vi "Configuration_old.vi"(10 "Open from\nscan VI":bool, 11 "Measurements":T1(tab)) -> (3 "configured?":bool)   [LabVIEW 2013]
uses:
  InstrControl/InstrumentSetup.vi
  InstrControl/InstrControl.lvclass
  globals/QC_MeasurementSetup.vi
  InstrControl/Switching/Switching.lvclass
  globals/QC_RunInformation.vi
panel:
  in  "Defaults Multimeter":bool
  in  "Multimeter":enum32{"Keithley 2000"}(tab)
  in  "Range Value\n(0.1 - 100)":dbl=100.0 format="%#.2g"
  in  "Range":u16(ring) items=["Auto", "Manual"]
  in  "Function":u16(ring)=3 items=["AC Current", "DC Current", "AC Voltage", "DC Voltage", "2W-Resistance", "4W-Resistance", "Period", "Frequency", "Temperature", "Diode", "Continuity"]
  in  "GPIB Address KE2000":i32=19
  in  "Apply":bool
  in  "Defaults LCR":bool
  in  "LCRs":enum32{"WayneKerr 6440B", "WayneKerr 6425"}(tab)
  in  "AC frequency [Hz]":i32=1000 format="%#.3p"
  in  "RC Configuration":u16(ring) items=["serial", "parallel"]
  in  "AC amplitude [V]":sgl=0.1
  in  "GPIB Address WK6440B":i32=23
  in  "GPIB Address WK6425":i32=17
  in  "AC amplitude [V] WK6425":sgl=0.1 caption="AC amplitude [V]"
  in  "RC Configuration WK6425":u16(ring) caption="RC Configuration" items=["serial", "parallel"]
  in  "AC frequency [Hz] WK6425":i32=1000 caption="AC frequency [Hz]" format="%#.3p"
  in  "VISA address":refnum<visa-resource-name>="COM24" caption="Arduino address"
  out "Programm uploaded?":string="Make sure programme is uploaded to Arduino Uno ->"
  in  "Blank Button":bool
  in  "Matrix address":i32=1
  in  "GPIB address":i32=10
  in  "Mux1 address":i32=4
  in  "Mux2 address":i32=5
  in  "Search Button":bool
  out "DIAGNOSTIC? Response":string
  out "Display Matrix":bool[][](array[boolean])
  in  "No Matrix":bool
  out "X Mapping":string[](array[string])
  out "Y Mapping":string[](array[string])
  in  "Change Preset Parameters":bool
  in  "V_breakdown Limit [V]":dbl=-500.0
  in  "IV Temperature Readout":enum16{"Read Arduino", "Enter manually"}(ring) caption="Temperature Readout"
  in  "IV Ramp down Interval [s]":i32=1 caption="Ramp down Interval [s]"
  in  "IV Ramp down steps [V]":dbl=50.0 caption="Ramp down steps [V]"
  in  "IV Step Interval [s]":i32=10 caption="Step Interval [s]"
  in  "IV Step Size [V]":dbl=10.0 caption="Step Size [V]" format="%.1f"
  in  "IV Final Voltage [V]":dbl=-700.0 caption="Final Voltage [V]" format="%.1f"
  in  "IV Initial Voltage [V]":dbl caption="Initial Voltage [V]" format="%.1f"
  in  "IV Voltage Supply":string(combo)="Keithley 2410"
  in  "Save IV defaults":bool
  in  "V_depletion Limit [V]":dbl=-300.0
  in  "CV LCR Meter":string(combo)="WayneKerr 6440B"
  in  "CV Temperature Readout":enum16{"Read Arduino", "Enter manually"}(ring) caption="Temperature Readout"
  in  "Save CV defaults":bool
  in  "CV Voltage Supply":string(combo)="Keithley 2410"
  in  "CV Initial Voltage [V]":dbl caption="Initial Voltage [V]" format="%.1f"
  in  "CV Final Voltage [V]":dbl=-700.0 caption="Final Voltage [V]" format="%.1f"
  in  "CV Step Size [V]":dbl=10.0 caption="Step Size [V]" format="%.1f"
  in  "CV Step Interval [s]":i32=5 caption="Step Interval [s]"
  in  "CV Ramp down steps [V]":dbl=10.0 caption="Ramp down steps [V]"
  in  "CV Ramp down Interval [s]":i32=1 caption="Ramp down Interval [s]"
  in  "Maximum current fluctuation [%]":dbl=2.0
  in  "Save Stability defaults":bool
  in  "Stability Voltage Supply":string(combo)="Keithley 487"
  in  "Fraction of good strips [%]":dbl=98.0
  in  "Bias Supply":string(combo)="Keithley 487"
  in  "SMU":string(combo)="Keithley 2410"
  in  "C_is Limit [pF/cm]":dbl=1.0
  in  "Save Cis defaults":bool
  in  "Cis Voltage Supply":string(combo)="Keithley 2410"
  in  "Cis Temperature Readout":enum16{"Read Arduino", "Enter manually"}(ring) caption="Temperature Readout"
  in  "Cis LCR Meter":string(combo)="WayneKerr 6440B"
  in  "Cis Ramp down Interval [s]":i32=1 caption="Ramp down Interval [s]"
  in  "Cis Ramp down steps [V]":dbl=50.0 caption="Ramp down steps [V]"
  in  "Cis Step Interval [s]":i32=10 caption="Step Interval [s]"
  in  "Cis Step Size [V]":dbl=10.0 caption="Step Size [V]" format="%.1f"
  in  "Cis Final Voltage [V]":dbl=-700.0 caption="Final Voltage [V]" format="%.1f"
  in  "Cis Initial Voltage [V]":dbl caption="Initial Voltage [V]" format="%.1f"
  in  "Ris Voltmeter":string(combo)="Keithley 2000"
  in  "Ris SMU":string(combo)="Keithley 6517"
  in  "Ris Bias Supply":string(combo)="Keithley 487"
  in  "Ris Temperature Readout":enum16{"Read Arduino", "Enter manually"}(ring) caption="Temperature Readout"
  in  "Save Ris defaults":bool
  in  "Ris Initial Voltage [V]":dbl caption="Initial Voltage [V]" format="%.1f"
  in  "Ris Final Voltage [V]":dbl=-700.0 caption="Final Voltage [V]" format="%.1f"
  in  "Ris Step Size [V]":dbl=10.0 caption="Step Size [V]" format="%.1f"
  in  "Ris Step Interval [s]":i32=10 caption="Step Interval [s]"
  in  "Ris Ramp down steps [V]":dbl=50.0 caption="Ramp down steps [V]"
  in  "Ris Ramp down Interval [s]":i32=1 caption="Ramp down Interval [s]"
  in  "R_is Limit [MOhm]":dbl=100.0
  in  "Supplies":T2(tab)
  in  "Current Limit [µA]":sgl=100.0
  in  "GPIB Address KE2410":i32=24
  in  "GPIB Address KE487":i32=22
  in  "Compliance":u16(ring) items=["20µA", "2mA"]
  in  "Range:":u16(ring) items=["Autorange", "2nA", "20nA", "200nA", "2 microAmp", "20 microAmp", "200 microAmp", "2 milliAmp"]
  in  "Current Limit":u16(ring)=1 items=["OFF", "ON"]
  in  "GPIB Address KE6517":i32=27
  in  "current compliance \nlevel [mA]":dbl=0.0001 format="%.4f"
  in  "compliance/\nmeasurement range (auto:0)":u16(ring)=6 items=["auto / auto", "1 nA / 1.1 V", "10 nA / 11 V", "100 nA / 110 V", "0.001 mA / 110 V", "0.01 mA / 110 V", "0.1 mA / 110 V", "1 mA / 110 V", "10 mA / 110 V", "100 mA / 110 V"]
  in  "GPIB Address KE236":i32=16
  in  "Defaults Supply":bool
  in  "OK Button":bool
  out "X Mapping CB Standard":string[](array[string])
  # "Measurement Configuration"
  # "MUX / Matrix Setup"
  # "Does not apply\nto striptest"
  # "Arduino Configuration"
  # "Multimeter Configuration"
  # "Supply Configuration"
  # "LCR Configuration"
  # "Only for\ninitialisation"
  # "Only for\ninitialisation"
  # "Does not do \nanything yet!"
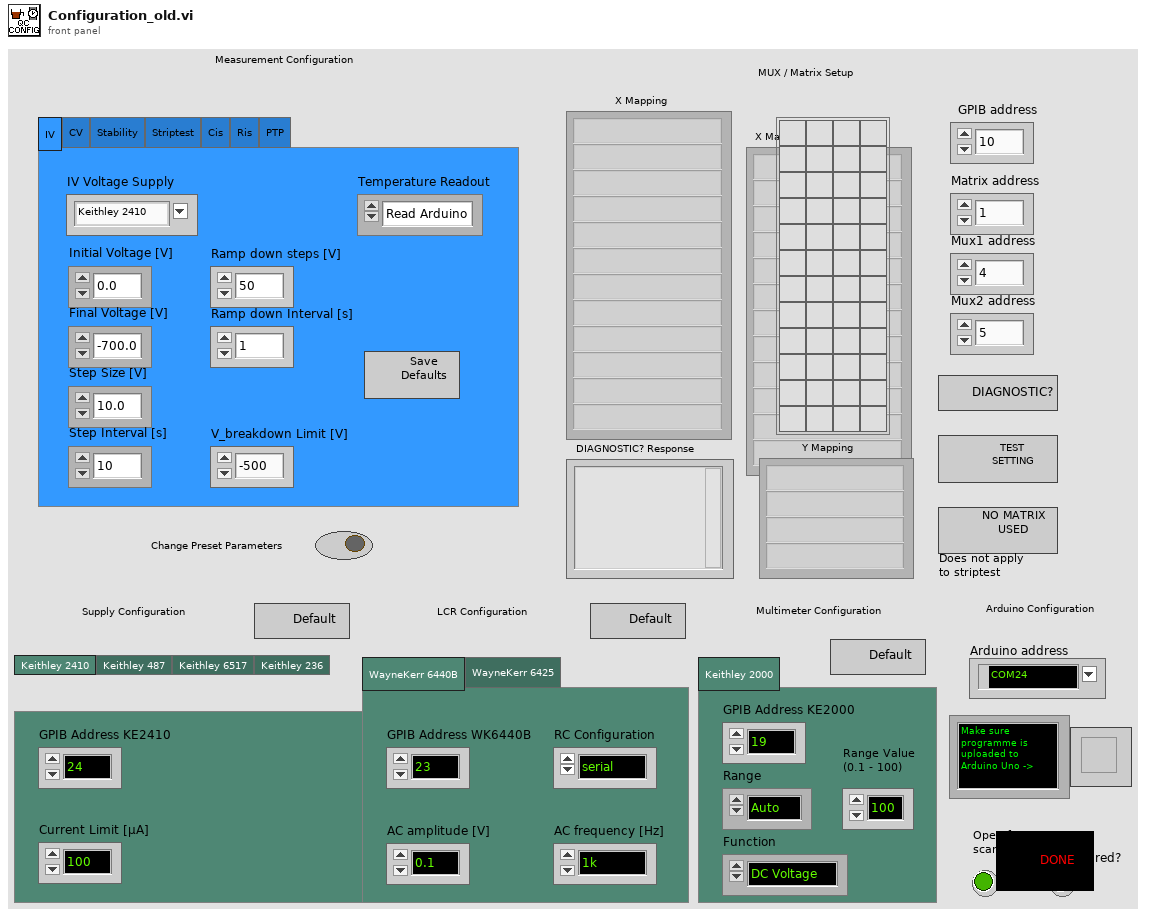
[diagram p1: front panel]
types:
  T1 = enum32{"IV", "CV", "Stability", "Striptest", "Cis", "Ris", "PTP"}
  T2 = enum32{"Keithley 2410", "Keithley 487", "Keithley 6517", "Keithley 236"}
  T3 = enum16{"Reset", "Ground", "Striptest SMU", "Striptest LCR", "IV", "CV", "Interstrip Cap", "Interstrip Res"}
  T4 = cluster{"Matrix address":string, "Mux1 address":string, "Mux2 address":string, "Matrix used?":bool, "Pickering":refnum<class "Pickering.lvclass">, "Matrix X Channels":cluster{"Bias Supply / SMU LO":i32, "Bias Supply / SMU HI":i32, "CV Box LO":i32, "CV Box HI":i32, "CV Box LO IN":i32, "CV Box HI IN":i32, "Volt meter LO":i32, "Volt meter HI":i32, "Mux1 C1":i32, "Mux1 C2":i32, "Mux2 C1":i32, "Mux2 C2":i32}}
  T5 = cluster{"Bias Supply":refnum<class "SupplyControl.lvclass">, "SMU":refnum<class "SupplyControl.lvclass">, "Multimeter":refnum<class "MultimeterControl.lvclass">, "Initial Voltage [V]":dbl, "Final Voltage [V]":dbl, "Step Size [V]":dbl, "Step Interval [s]":i32, "Number Of Steps":u32, "Ramp down steps [V]":dbl, "Ramp down Interval [s]":i32, "Set Current Limit?":bool, "Current Limit [µA]":dbl, "Temperature Readout":enum16{"Read Arduino", "Enter manually"}, "Arduino":refnum<class "ArduinoControl.lvclass">, "Supply Name":string, "SMU Name":string, "Voltmeter Name":string, "R_is Limit [MOhm]":dbl, "Switching":refnum<class "Switching.lvclass">, "Matrix used?":bool, "Matrix X Channels":cluster{"Bias Supply / SMU LO":i32, "Bias Supply / SMU HI":i32, "CV Box LO":i32, "CV Box HI":i32, "CV Box LO IN":i32, "CV Box HI IN":i32, "Volt meter LO":i32, "Volt meter HI":i32, "Mux1 C1":i32, "Mux1 C2":i32, "Mux2 C1":i32, "Mux2 C2":i32}}
  T6 = cluster{"Supply":refnum<class "SupplyControl.lvclass">, "LCR":refnum<class "LCRControl.lvclass">, "Initial Voltage [V]":dbl, "Final Voltage [V]":dbl, "Step Size [V]":dbl, "Step Interval [s]":i32, "Number Of Steps":u32, "AC frequency [Hz]":i32, "RC Configuration":u16, "AC amplitude [V]":dbl, "Ramp down steps [V]":dbl, "Ramp down Interval [s]":i32, "Set Current Limit?":bool, "Current Limit [µA]":dbl, "Temperature Readout":enum16{"Read Arduino", "Enter manually"}, "Arduino":refnum<class "ArduinoControl.lvclass">, "Supply Name":string, "LCR Name":string, "V_depletion Limit [V]":dbl, "Switching":refnum<class "Switching.lvclass">, "Matrix used?":bool, "Matrix X Channels":cluster{"Bias Supply / SMU LO":i32, "Bias Supply / SMU HI":i32, "CV Box LO":i32, "CV Box HI":i32, "CV Box LO IN":i32, "CV Box HI IN":i32, "Volt meter LO":i32, "Volt meter HI":i32, "Mux1 C1":i32, "Mux1 C2":i32, "Mux2 C1":i32, "Mux2 C2":i32}}
  T7 = cluster{"Supply":refnum<class "SupplyControl.lvclass">, "LCR":refnum<class "LCRControl.lvclass">, "Initial Voltage [V]":dbl, "Final Voltage [V]":dbl, "Step Size [V]":dbl, "Step Interval [s]":i32, "Number Of Steps":u32, "AC frequency [Hz]":i32, "RC Configuration":u16, "AC amplitude [V]":dbl, "Ramp down steps [V]":dbl, "Ramp down Interval [s]":i32, "Set Current Limit?":bool, "Current Limit [µA]":dbl, "Temperature Readout":enum16{"Read Arduino", "Enter manually"}, "Arduino":refnum<class "ArduinoControl.lvclass">, "Supply Name":string, "LCR Name":string, "C_is Limit [pF/cm]":dbl, "Switching":refnum<class "Switching.lvclass">, "Matrix used?":bool, "Matrix X Channels":cluster{"Bias Supply / SMU LO":i32, "Bias Supply / SMU HI":i32, "CV Box LO":i32, "CV Box HI":i32, "CV Box LO IN":i32, "CV Box HI IN":i32, "Volt meter LO":i32, "Volt meter HI":i32, "Mux1 C1":i32, "Mux1 C2":i32, "Mux2 C1":i32, "Mux2 C2":i32}}
  T8 = cluster{"Supply":refnum<class "SupplyControl.lvclass">, "Initial Voltage [V]":dbl, "Final Voltage [V]":dbl, "Step Size [V]":dbl, "Step Interval [s]":i32, "Number Of Steps":u32, "Ramp down steps [V]":dbl, "Ramp down Interval [s]":i32, "hold steps":i32, "Set Current Limit?":bool, "Current Limit [µA]":dbl, "Temperature Readout":enum16{"Read Arduino", "Enter manually"}, "Arduino":refnum<class "ArduinoControl.lvclass">, "Supply Name":string, "V_breakdown Limit [V]":dbl, "Switching":refnum<class "Switching.lvclass">, "Matrix used?":bool, "Matrix X Channels":cluster{"Bias Supply / SMU LO":i32, "Bias Supply / SMU HI":i32, "CV Box LO":i32, "CV Box HI":i32, "CV Box LO IN":i32, "CV Box HI IN":i32, "Volt meter LO":i32, "Volt meter HI":i32, "Mux1 C1":i32, "Mux1 C2":i32, "Mux2 C1":i32, "Mux2 C2":i32}}
  T9 = cluster{"VISA address":refnum<visa-resource-name>, "T sensor":enum16{"SHT", "DS"}, "Arduino":refnum<class "ArduinoControl.lvclass">}
  T10 = cluster{"Range":u16, "Range Value":dbl, "Function":u16, "KE2000":refnum<class "KE2000.lvclass">}
  T11 = enum16{"Left Button", "Center Button", "Right Button", "Window Close"}
  T12 = cluster{"Sensor Serial No.:":string, "Wafer Serial No.:":string, "Batch:":string, "Manufacturer:":string, "Device Category:":string, "Database Serial No.:":string, "Date Initiated:":string, "Time Initiated:":string, "Test":string, "Instruments used:":string, "Probeplan used:":string, "End of Run comment:":string, "User:":string}
  T13 = cluster{"RC Configuration":u16, "AC amplitude [V]":dbl, "AC frequency [Hz]":i32, "WK6440B":refnum<class "WK6440B.lvclass">}
  T14 = cluster{"RC Configuration":u16, "AC amplitude [V]":dbl, "AC frequency [Hz]":i32, "WK6425":refnum<class "WK6425.lvclass">}
  T15 = cluster{"Current Limit":sgl, "KE2410":refnum<class "KE2410.lvclass">}
  T16 = cluster{"Compliance":u16, "Range:":u16, "KE487":refnum<class "KE487.lvclass">}
  T17 = cluster{"Current Limit":u16, "KE6517":refnum<class "KE6517.lvclass">}
  T18 = cluster{"current \ncompliance level":dbl, "compliance/\nmeasurement range (auto:0)":u16, "KE236":refnum<class "KE236.lvclass">}
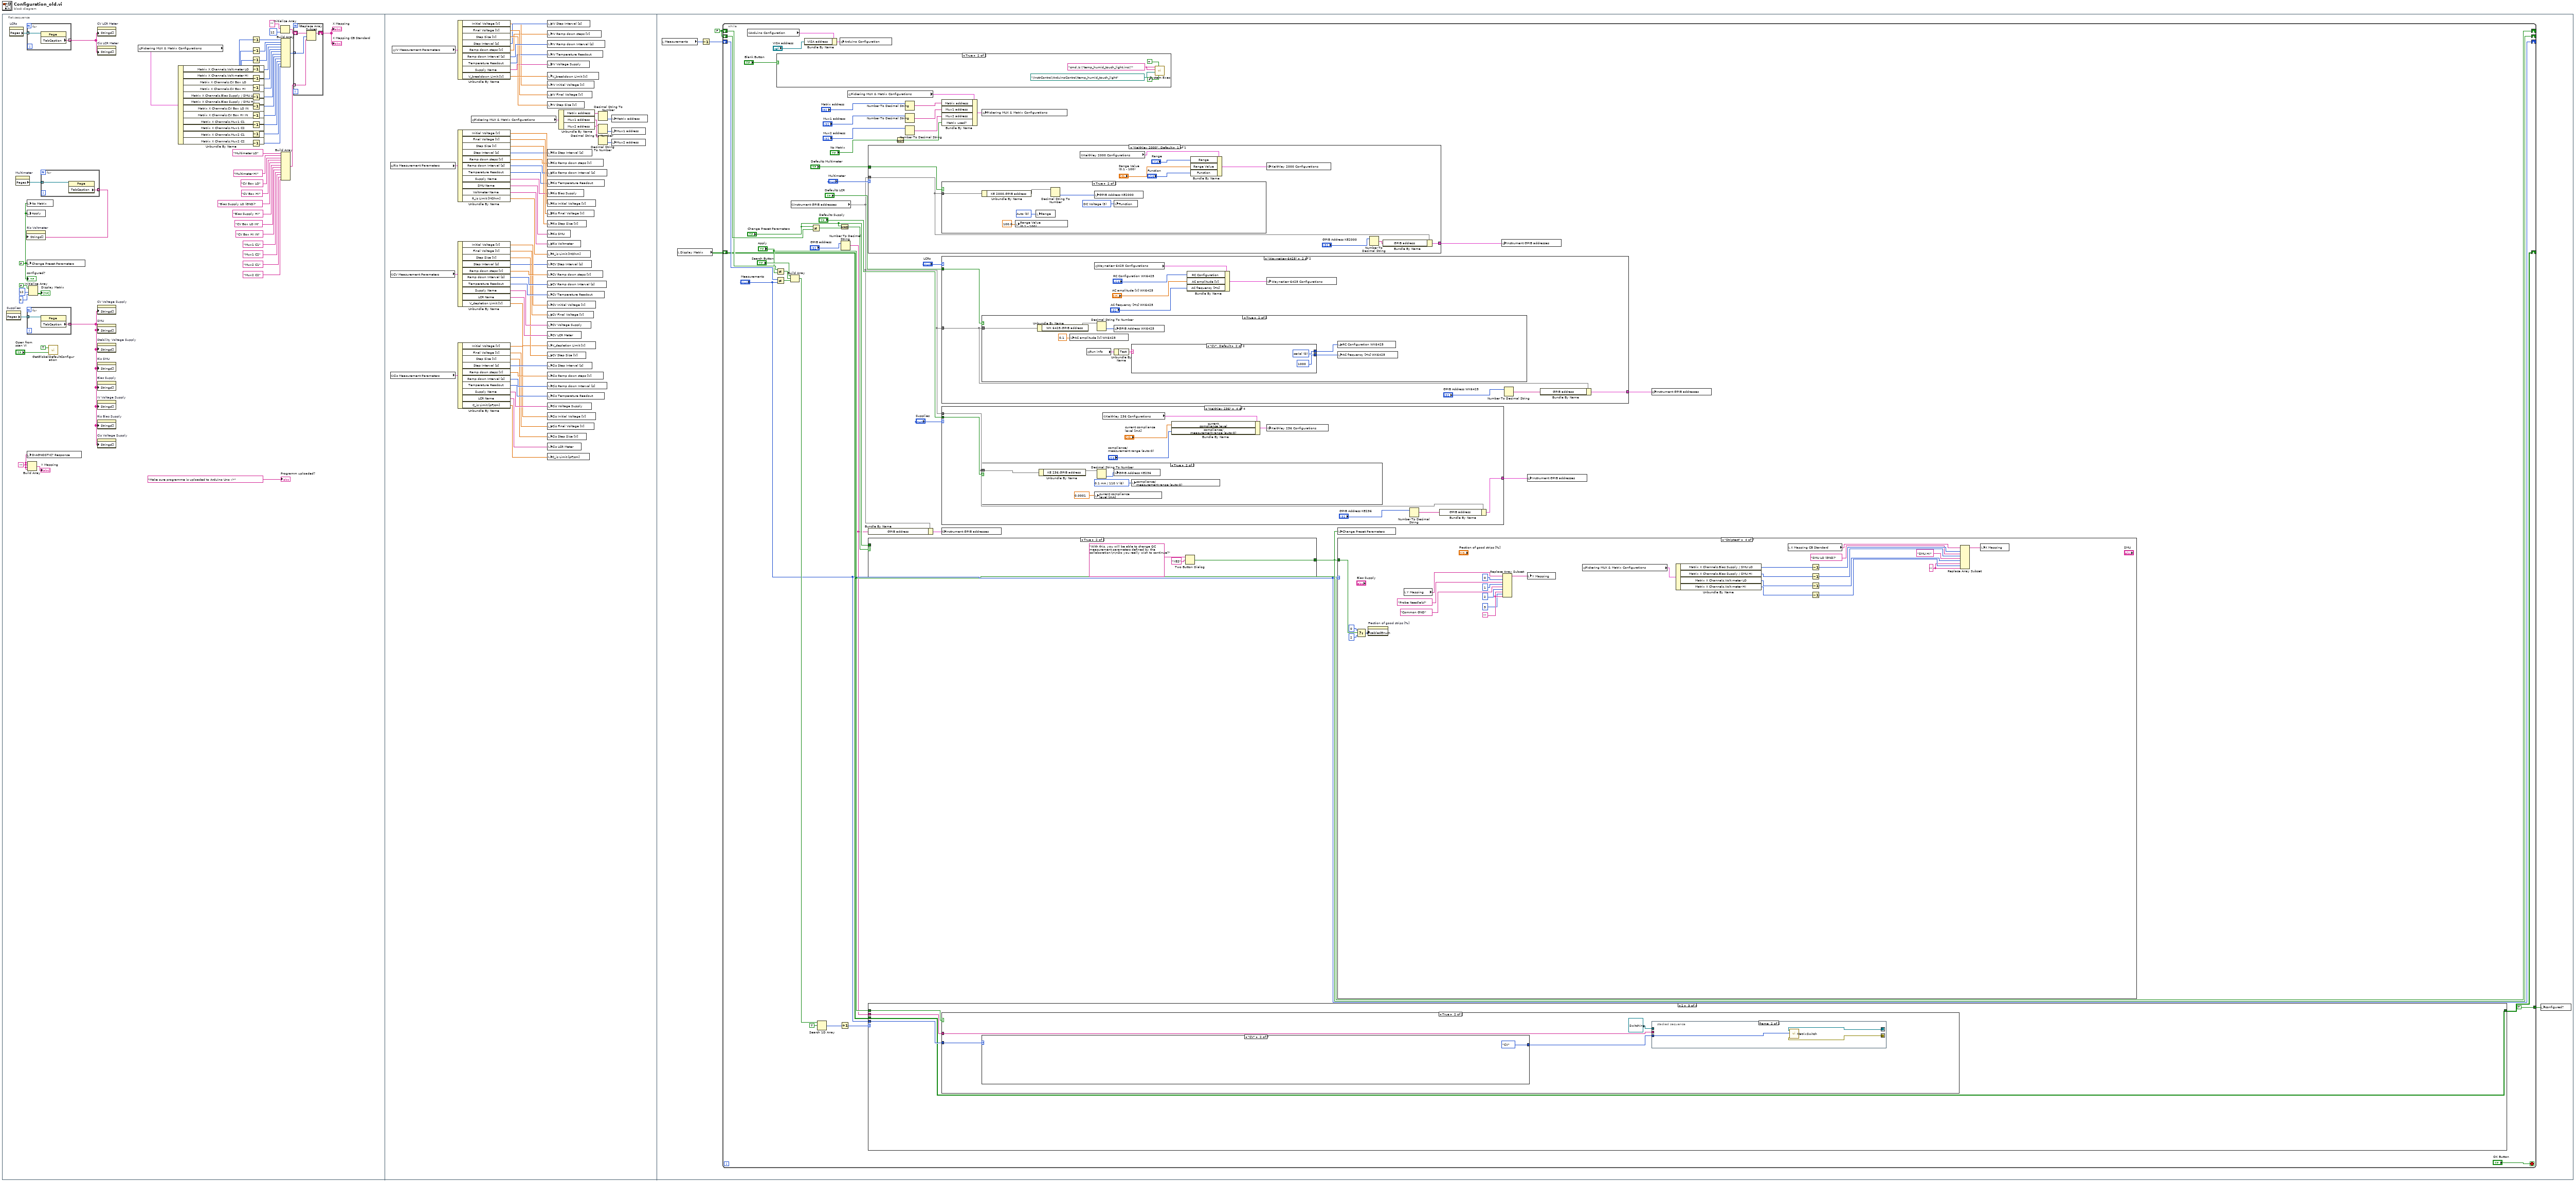
[diagram p0: block diagram]
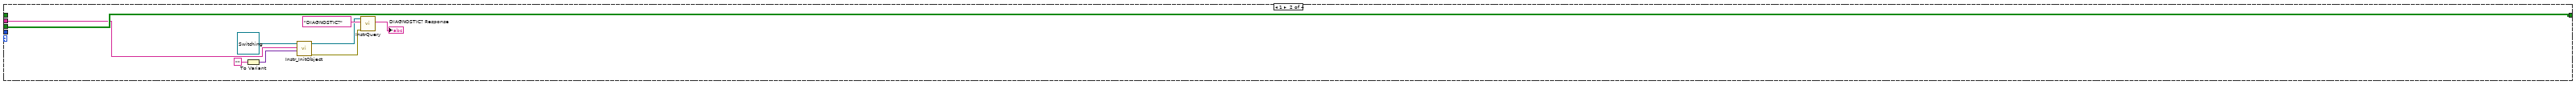
[diagram p3: hidden frame]
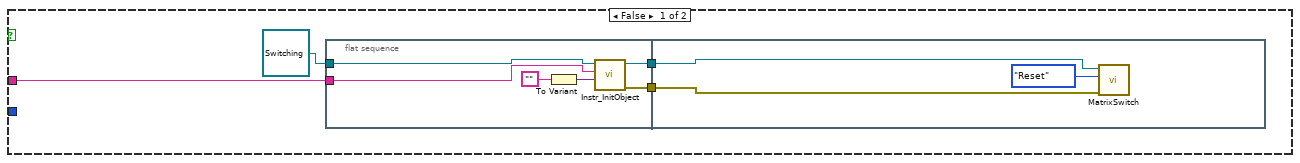
[diagram p4: hidden frame]
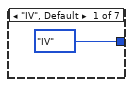
[diagram p5: hidden frame]
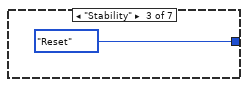
[diagram p6: hidden frame]
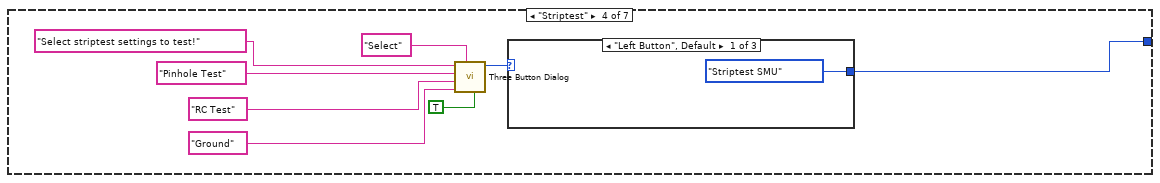
[diagram p7: hidden frame]
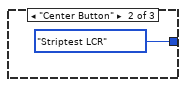
[diagram p8: hidden frame]
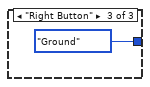
[diagram p9: hidden frame]
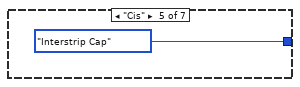
[diagram p10: hidden frame]
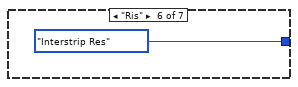
[diagram p11: hidden frame]
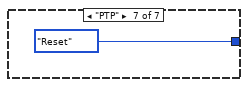
[diagram p12: hidden frame]
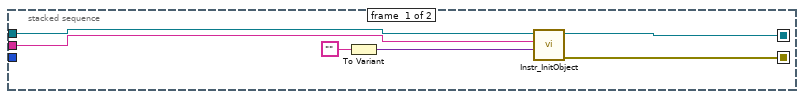
[diagram p13: hidden frame]
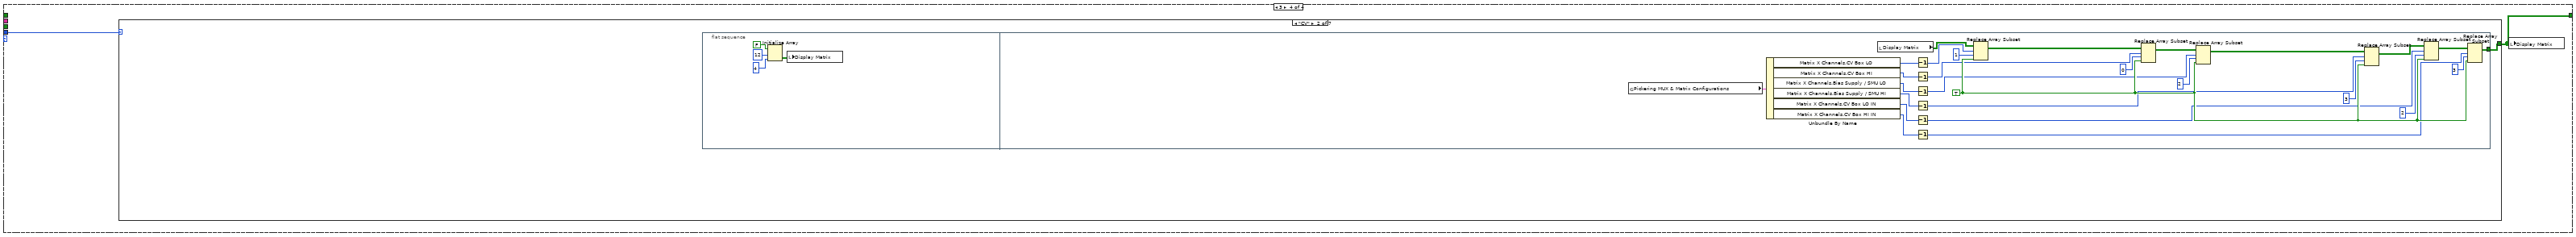
[diagram p14: hidden frame]
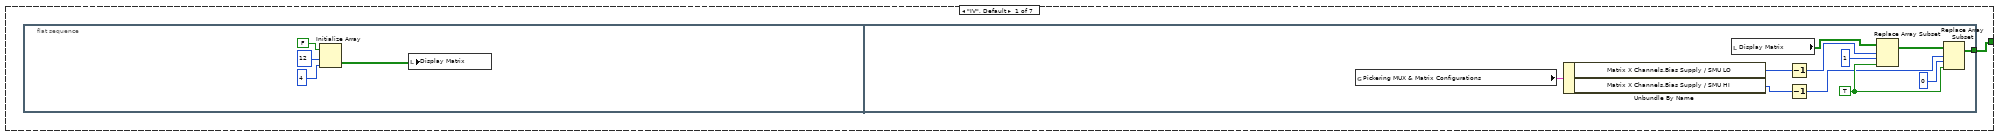
[diagram p15: hidden frame]
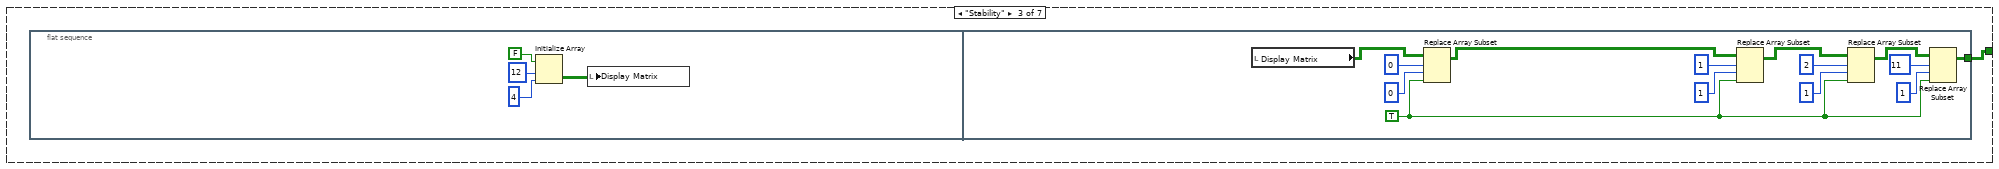
[diagram p16: hidden frame]
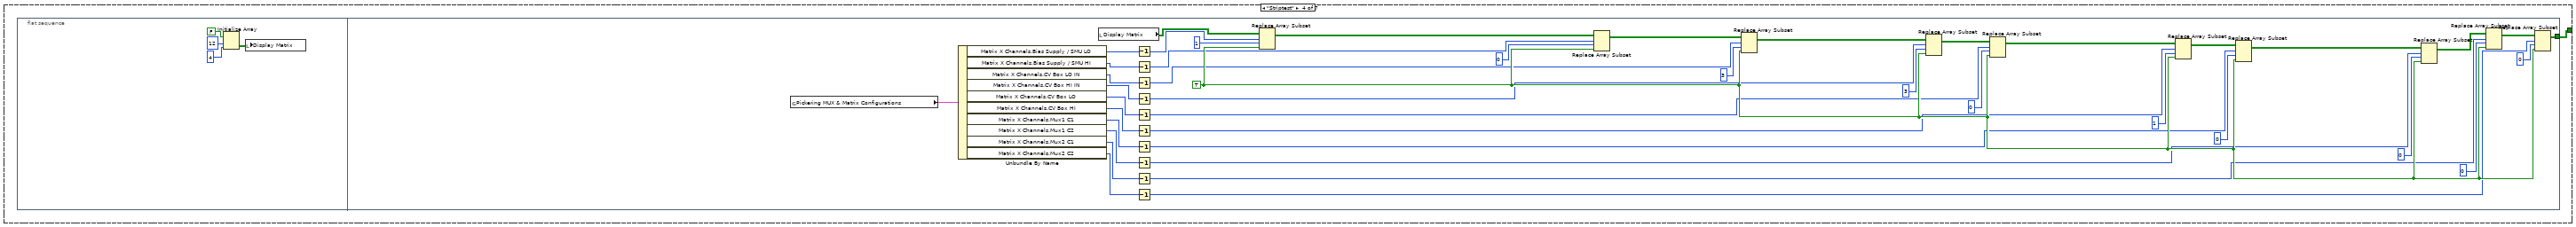
[diagram p17: hidden frame]
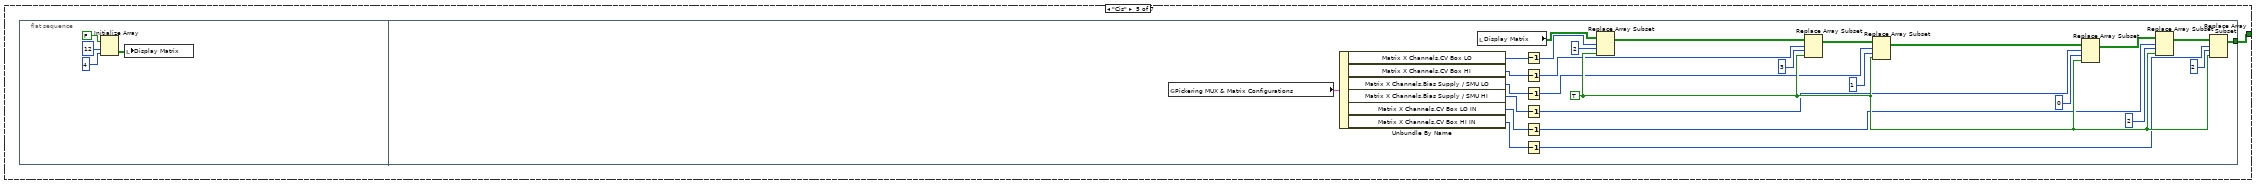
[diagram p18: hidden frame]
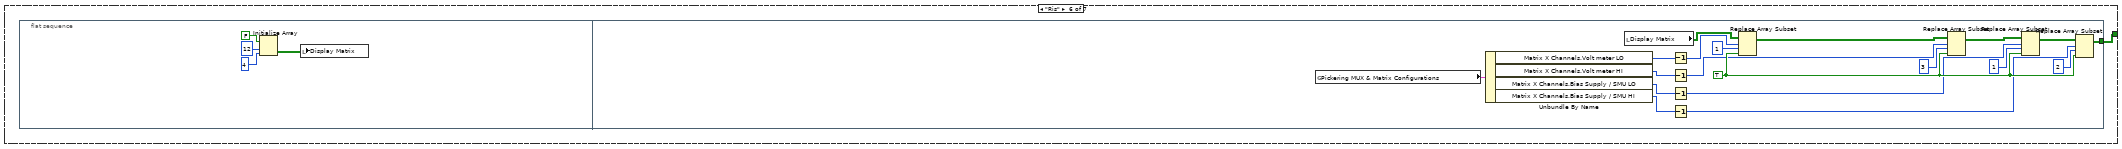
[diagram p19: hidden frame]
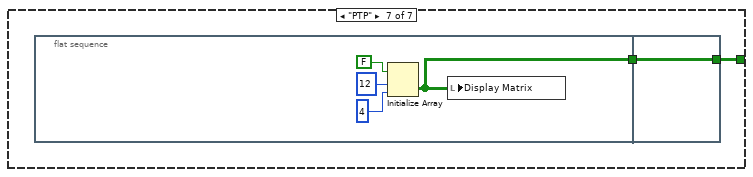
[diagram p20: hidden frame]
diagram:
  n1 = flat-sequence {
    frame #0 {
      w42 = FALSE
      w41 = ""
      n2 = property on="Supplies" class="TabCtl (strict)"() -> ("Pages"=w45:refnum<vi>[])  [unwired: 2 in, 2 out]
      n3 = property on="LCRs" class="TabCtl (strict)"() -> ("Pages"=w44:refnum<vi>[])  [unwired: 2 in, 2 out]
      n4 = property on="Multimeter" class="TabCtl (strict)"() -> ("Pages"=w40:refnum<vi>[])  [unwired: 2 in, 2 out]
      n5 = for {
        tunnel: w44 -> [w67] mode=indexing
        tunnel: [w66] -> w43 mode=indexing
        n6 = property class="Page"(reference=w67) -> ("TabCaption"=w66:string)  [unwired: 1 in, 2 out]
      }
      n7 = local write "No Matrix"(w42) -> ()
      n8 = local write "Apply"(w42) -> ()
      n9 = local write "Change Preset Parameters"(w42) -> ()
      n10 = for {
        tunnel: w45 -> [w69] mode=indexing
        tunnel: [w68] -> w38 mode=indexing
        n11 = property class="Page"(reference=w69) -> ("TabCaption"=w68:string)  [unwired: 1 in, 2 out]
      }
      n12 = local write "DIAGNOSTIC? Response"(w41) -> ()
      n13 = Build Array(w41, w41, w41, w41) -> (→"Y Mapping":string[])
      n14 = Initialize Array(FALSE, 12, 4) -> (→"Display Matrix":bool[][])
      n15 = for {
        tunnel: w40 -> [w65] mode=indexing
        tunnel: [w64] -> w39 mode=indexing
        n16 = property class="Page"(reference=w65) -> ("TabCaption"=w64:string)  [unwired: 1 in, 2 out]
      }
      n17 = property on="Ris Voltmeter" class="CmbBox"("Strings[]"=w39) -> ()  [unwired: 2 in, 2 out]
      n18 = call "GetGlobalDefaultConfiguration.vi"("DO NOT override instruments"="Open from\nscan VI", "Read defaults?"=TRUE) -> ()  [unwired: 1 in, 1 out]
      n19 = property on="CV LCR Meter" class="CmbBox"("Strings[]"=w43) -> ()  [unwired: 2 in, 2 out]
      n20 = property on="Cis LCR Meter" class="CmbBox"("Strings[]"=w43) -> ()  [unwired: 2 in, 2 out]
      n21 = property on="CV Voltage Supply" class="CmbBox"("Strings[]"=w38) -> ()  [unwired: 2 in, 2 out]
      n22 = property on="SMU" class="CmbBox"("Strings[]"=w38) -> ()  [unwired: 2 in, 2 out]
      n23 = property on="Stability Voltage Supply" class="CmbBox"("Strings[]"=w38) -> ()  [unwired: 2 in, 2 out]
      n24 = property on="Ris SMU" class="CmbBox"("Strings[]"=w38) -> ()  [unwired: 2 in, 2 out]
      n25 = property on="Bias Supply" class="CmbBox"("Strings[]"=w38) -> ()  [unwired: 2 in, 2 out]
      n26 = property on="IV Voltage Supply" class="CmbBox"("Strings[]"=w38) -> ()  [unwired: 2 in, 2 out]
      n27 = property on="Ris Bias Supply" class="CmbBox"("Strings[]"=w38) -> ()  [unwired: 2 in, 2 out]
      n28 = property on="Cis Voltage Supply" class="CmbBox"("Strings[]"=w38) -> ()  [unwired: 2 in, 2 out]
      n29 = global read "InstrumentSetup.vi" "Pickering MUX & Matrix Configurations"() -> (w31:T4)
      n30 = Unbundle By Name(w31) -> ("Matrix X Channels.Volt meter LO"=w20:i32, "Matrix X Channels.Volt meter HI"=w18:i32, "Matrix X Channels.CV Box LO"=w30:i32, "Matrix X Channels.CV Box HI"=w25:i32, "Matrix X Channels.Bias Supply / SMU LO"=w26:i32, "Matrix X Channels.Bias Supply / SMU HI"=w27:i32, "Matrix X Channels.CV Box LO IN"=w28:i32, "Matrix X Channels.CV Box HI IN"=w29:i32, "Matrix X Channels.Mux1 C1"=w21:i32, "Matrix X Channels.Mux1 C2"=w22:i32, "Matrix X Channels.Mux2 C1"=w23:i32, "Matrix X Channels.Mux2 C2"=w24:i32)
      n31 = Decrement(x=w20) -> (x-1=w19:i32)
      n32 = Decrement(x=w18) -> (x-1=w17:i32)
      n33 = Decrement(x=w30) -> (x-1=w16:i32)
      n34 = Decrement(x=w25) -> (x-1=w15:i32)
      n35 = Decrement(x=w26) -> (x-1=w14:i32)
      n36 = Decrement(x=w27) -> (x-1=w13:i32)
      n37 = Decrement(x=w28) -> (x-1=w12:i32)
      n38 = Decrement(x=w29) -> (x-1=w11:i32)
      n39 = Decrement(x=w21) -> (x-1=w10:i32)
      n40 = Decrement(x=w22) -> (x-1=w9:i32)
      n41 = Decrement(x=w23) -> (x-1=w8:i32)
      n42 = Decrement(x=w24) -> (x-1=w7:i32)
      n43 = Initialize Array("", 12) -> (w2:string[])
      n44 = Build Array(w19, w17, w16, w15, w14, w13, w12, w11, w10, w9, w8, w7) -> (w6:i32[])
      n45 = Build Array("Multimeter LO" ("Input Element"), "Multimeter HI" ("Input Element"), "CV Box LO" ("Input Element"), "CV Box HI" ("Input Element"), "Bias Supply LO (GND)" ("Input Element"), "Bias Supply HI" ("Input Element"), "CV Box LO IN" ("Input Element"), "CV Box HI IN" ("Input Element"), "Mux1 C1" ("String"), "Mux1 C2" ("String"), "Mux2 C1" ("String"), "Mux2 C2" ("String")) -> (w5:string[])
      n46 = for {
        tunnel: w6 -> [w61] mode=indexing
        tunnel: w5 -> [w62] mode=indexing
        shift-right: [w60] -> w1
        shift-left: w2 -> [w63]
        n47 = Replace Array Subset(array=w63, new element=w62, index=w61) -> (w60:string[])
      }
      "X Mapping" <- w1
      "X Mapping CB Standard" <- w1
      "configured?" <- w42
      "Programm uploaded?" <- "Make sure programme is uploaded to Arduino Uno ->"
    }
    frame #1 {
      n48 = global read "QC_MeasurementSetup.vi" "Ris Measurement Parameters"() -> (w81:T5)
      n49 = global read "QC_MeasurementSetup.vi" "CV Measurement Parameters"() -> (w82:T6)
      n50 = global read "QC_MeasurementSetup.vi" "Cis Measurement Parameters"() -> (w93:T7)
      n51 = global read "QC_MeasurementSetup.vi" "IV Measurement Parameters"() -> (w111:T8)
      n52 = Unbundle By Name(w111) -> ("Initial Voltage [V]"=w112:dbl, "Final Voltage [V]"=w117:dbl, "Step Size [V]"=w118:dbl, "Step Interval [s]"=w114:i32, "Ramp down steps [V]"=w113:dbl, "Ramp down Interval [s]"=w120:i32, "Temperature Readout"=w115:enum16{"Read Arduino", "Enter manually"}, "Supply Name"=w116:string, "V_breakdown Limit [V]"=w119:dbl)
      n53 = Unbundle By Name(w81) -> ("Initial Voltage [V]"=w80:dbl, "Final Voltage [V]"=w79:dbl, "Step Size [V]"=w73:dbl, "Step Interval [s]"=w72:i32, "Ramp down steps [V]"=w76:dbl, "Ramp down Interval [s]"=w78:i32, "Temperature Readout"=w71:enum16{"Read Arduino", "Enter manually"}, "Supply Name"=w77:string, "SMU Name"=w75:string, "Voltmeter Name"=w74:string, "R_is Limit [MOhm]"=w70:dbl)
      n54 = Unbundle By Name(w82) -> ("Initial Voltage [V]"=w85:dbl, "Final Voltage [V]"=w86:dbl, "Step Size [V]"=w87:dbl, "Step Interval [s]"=w84:i32, "Ramp down steps [V]"=w88:dbl, "Ramp down Interval [s]"=w92:i32, "Temperature Readout"=w91:enum16{"Read Arduino", "Enter manually"}, "Supply Name"=w89:string, "LCR Name"=w90:string, "V_depletion Limit [V]"=w83:dbl)
      n55 = Unbundle By Name(w93) -> ("Initial Voltage [V]"=w94:dbl, "Final Voltage [V]"=w95:dbl, "Step Size [V]"=w96:dbl, "Step Interval [s]"=w98:i32, "Ramp down steps [V]"=w97:dbl, "Ramp down Interval [s]"=w99:i32, "Temperature Readout"=w100:enum16{"Read Arduino", "Enter manually"}, "Supply Name"=w101:string, "LCR Name"=w102:string, "C_is Limit [pF/cm]"=w103:dbl)
      n56 = global read "InstrumentSetup.vi" "Pickering MUX & Matrix Configurations"() -> (w110:T4)
      n57 = local write "IV Step Interval [s]"(w114) -> ()
      n58 = local write "IV Ramp down steps [V]"(w113) -> ()
      n59 = local write "IV Ramp down Interval [s]"(w120) -> ()
      n60 = local write "IV Temperature Readout"(w115) -> ()
      n61 = local write "IV Voltage Supply"(w116) -> ()
      n62 = local write "V_breakdown Limit [V]"(w119) -> ()
      n63 = local write "IV Initial Voltage [V]"(w112) -> ()
      n64 = local write "IV Final Voltage [V]"(w117) -> ()
      n65 = local write "IV Step Size [V]"(w118) -> ()
      n66 = local write "Ris Step Interval [s]"(w72) -> ()
      n67 = local write "Ris Ramp down steps [V]"(w76) -> ()
      n68 = local write "Ris Ramp down Interval [s]"(w78) -> ()
      n69 = local write "Ris Temperature Readout"(w71) -> ()
      n70 = local write "Ris Bias Supply"(w77) -> ()
      n71 = local write "Ris Initial Voltage [V]"(w80) -> ()
      n72 = local write "Ris Final Voltage [V]"(w79) -> ()
      n73 = local write "Ris Step Size [V]"(w73) -> ()
      n74 = local write "Ris SMU"(w75) -> ()
      n75 = local write "Ris Voltmeter"(w74) -> ()
      n76 = local write "R_is Limit [MOhm]"(w70) -> ()
      n77 = local write "CV Step Interval [s]"(w84) -> ()
      n78 = local write "CV Ramp down steps [V]"(w88) -> ()
      n79 = local write "CV Ramp down Interval [s]"(w92) -> ()
      n80 = local write "CV Temperature Readout"(w91) -> ()
      n81 = local write "CV Initial Voltage [V]"(w85) -> ()
      n82 = local write "CV Final Voltage [V]"(w86) -> ()
      n83 = local write "CV Voltage Supply"(w89) -> ()
      n84 = local write "CV LCR Meter"(w90) -> ()
      n85 = local write "V_depletion Limit [V]"(w83) -> ()
      n86 = local write "CV Step Size [V]"(w87) -> ()
      n87 = local write "Cis Step Interval [s]"(w98) -> ()
      n88 = local write "Cis Ramp down steps [V]"(w97) -> ()
      n89 = local write "Cis Ramp down Interval [s]"(w99) -> ()
      n90 = local write "Cis Temperature Readout"(w100) -> ()
      n91 = local write "Cis Voltage Supply"(w101) -> ()
      n92 = local write "Cis Initial Voltage [V]"(w94) -> ()
      n93 = local write "Cis Final Voltage [V]"(w95) -> ()
      n94 = local write "Cis Step Size [V]"(w96) -> ()
      n95 = local write "Cis LCR Meter"(w102) -> ()
      n96 = local write "C_is Limit [pF/cm]"(w103) -> ()
      n97 = Unbundle By Name(w110) -> ("Matrix address"=w109:string, "Mux1 address"=w108:string, "Mux2 address"=w104:string)
      n98 = Decimal String To Number(string=w109) -> (number=w106:i32)  [unwired: 2 in, 1 out]
      n99 = Decimal String To Number(string=w108) -> (number=w105:i32)  [unwired: 2 in, 1 out]
      n100 = Decimal String To Number(string=w104) -> (number=w107:i32)  [unwired: 2 in, 1 out]
      n101 = local write "Matrix address"(w106) -> ()
      n102 = local write "Mux1 address"(w105) -> ()
      n103 = local write "Mux2 address"(w107) -> ()
    }
    frame #2 {
      w122 = FALSE
      n104 = local read "Measurements"() -> (w124:T1)
      n105 = local read "Display Matrix"() -> (w121:bool[][])
      n106 = Decrement(x=w124) -> (x-1=w123:T1)
      n107 = while {
        shift-right: [w166] -> _
        shift-left: w122 -> [w169]
        shift-right: ["Measurements"] -> _
        shift-left: w123 -> [w154]
        shift-right: [w133] -> _
        shift-left: w121 -> [w132]
        tunnel: [TRUE] -> w125
        shift-right: ["Apply"] -> _
        shift-left: w122 -> [w148]
        stop <- "OK Button" stop-if-true
        n108 = global read "InstrumentSetup.vi" "Arduino Configuration"() -> (w152:T9)
        n109 = Not Equal?(x=w148, y="Apply") -> (x != y?=w138:bool)
        n110 = Not Equal?(x=w154, y="Measurements") -> (x != y?=w134:bool)
        n111 = case shown="True" "Blank Button" {
          frame False {
          }
          frame True {
            w471 = "cmd /c \"temp_humid_touch_light.ino\""
            n112 = call <vilib>:"System Exec.vi"("run minimized? (F)"=FALSE, "wait until completion? (T)"=TRUE, "working directory"=path "../InstrControl/ArduinoControl/temp_humid_touch_light", "standard input"=w471, "command line"=w471) -> ()  [unwired: 3 in, 4 out]
          }
        }
        n113 = Build Array("Search Button", w138, w134) -> (w140:bool[])
        n114 = global read "InstrumentSetup.vi" "Instrument GPIB addresses"() -> (w128)
        n115 = Bundle By Name(cluster=w152, "VISA address"="VISA address") -> (w153:T9)
        n116 = Not Equal?(x="Change Preset Parameters", y=w169) -> (x != y?=w168:bool)
        n117 = Search 1D Array(1D array=w140, element=TRUE) -> (index of element=w142:i32)  [unwired: 1 in]
        n118 = global write "InstrumentSetup.vi" "Arduino Configuration"(w153) -> ()
        n119 = And(x="Change Preset Parameters", y=w168) -> (x .and. y?=w170:bool)
        n120 = Increment(x=w142) -> (x+1=w139:i32)
        n121 = Number To Decimal String(number="GPIB address") -> (decimal integer string=w126:string)  [unwired: 1 in]
        n122 = global read "InstrumentSetup.vi" "Pickering MUX & Matrix Configurations"() -> (w157:T4)
        n123 = case shown="\"Keithley 2000\", Default" "Multimeter" {
          tunnel: "Defaults Multimeter" -> [w419]
          tunnel: w128 -> [w411]
          tunnel: [w410] -> w129
          frame "Keithley 2000", Default {
            n124 = case shown="True" w419 {
              tunnel: w411 -> [_ w425]
              frame False {
              }
              frame True {
                w421 = u16 0 items=["Auto", "Manual"] ("Range")
                w422 = u16 3 items=["AC Current", "DC Current", "AC Voltage", "DC Voltage", "2W-Resistance", "4W-Resistance", "Period", "Frequency", "Temperature", "Diode", "Continuity"] ("Function")
                n125 = Unbundle By Name(w425) -> ("KE 2000.GPIB address"=w424)
                n126 = local write "Range Value\n(0.1 - 100)"(100.0 ("Range Value\n(0.1 - 100)")) -> ()
                n127 = local write "Range"(w421) -> ()
                n128 = Decimal String To Number(string=w424) -> (number=w423:i32)  [unwired: 2 in, 1 out]
                n129 = local write "GPIB Address KE2000"(w423) -> ()
                n130 = local write "Function"(w422) -> ()
              }
            }
            n131 = global read "InstrumentSetup.vi" "Keithley 2000 Configurations"() -> (w418:T10)
            n132 = Bundle By Name(cluster=w418, "Range"="Range", "Range Value"="Range Value\n(0.1 - 100)", "Function"="Function") -> (w417:T10)
            n133 = global write "InstrumentSetup.vi" "Keithley 2000 Configurations"(w417) -> ()
            n134 = Number To Decimal String(number="GPIB Address KE2000") -> (decimal integer string=w412:string)  [unwired: 1 in]
            n135 = Bundle By Name(cluster=w411, "GPIB address"=w412) -> (w410:cluster{})
          }
        }
        n136 = Bundle By Name(cluster=w128, "GPIB address"=w126) -> (w127:cluster{})
        n137 = case shown="True" w170 {
          tunnel: [w474 w475] -> w166
          tunnel: "Change Preset Parameters" -> [w474 _]
          frame False {
          }
          frame True {
            n138 = Two Button Dialog(message="With this, you will be able to change QC measurement parameters defined by the collaboration!\n\nDo you really wish to continue?", 2:"YES") -> (T button?=w475:bool)  [unwired: 1 in]
          }
        }
        n139 = case shown="2" w139 {
          tunnel: "Measurements" -> [_ _ w185 w231]
          tunnel: "Apply" -> [_ _ w186 _]
          tunnel: [w173 w180 w184 w230] -> w133
          tunnel: w132 -> [w173 w180 w184 _]
          tunnel: w126 -> [_ w176 w183 _]
          frame 0, Default {
          }
          frame 1 {
            n140 = To Variant(anything="") -> (Variant=w174:variant)
            n141 = call-dynamic "Instr_InitObject.vi"("Instrument Configuration"=w174, "Instrument address"=w176, "Switching in"=refnum<class "Switching.lvclass"> refnum ("Switching.lvclass")) -> ("error out"=w177:errorcluster, "Switching out"=w178:refnum<class "Switching.lvclass">)  [unwired: 7 in]
            n142 = call-dynamic "InstrQuery.vi"("error in (no error)"=w177, "Command string"="DIAGNOSTIC?", "InstControl in"=w178) -> ("Instrument response"=→"DIAGNOSTIC? Response":string)  [unwired: 6 in, 2 out]
          }
          frame 2 {
            n143 = case shown="True" w186 {
              tunnel: w185 -> [_ w202]
              tunnel: w183 -> [w187 w200]
              frame False {
                n144 = flat-sequence {
                  tunnel: refnum<class "Switching.lvclass"> refnum ("Switching in") -> [w196]
                  tunnel: [w194] -> w189
                  tunnel: [w193] -> w188
                  tunnel: w187 -> [w195]
                  tunnel: w189 -> [w199]
                  tunnel: w188 -> [w198]
                  frame #0 {
                    n145 = To Variant(anything="") -> (Variant=w192:variant)
                    n146 = call-dynamic "Instr_InitObject.vi"("Instrument Configuration"=w192, "Instrument address"=w195, "Switching in"=w196) -> ("error out"=w193:errorcluster, "Switching out"=w194:refnum<class "Switching.lvclass">)  [unwired: 7 in]
                  }
                  frame #1 {
                    n147 = call-dynamic "MatrixSwitch.vi"("error in (no error)"=w198, "Action"=T3."Reset", "Switching in"=w199) -> ()  [unwired: 6 in, 3 out]
                  }
                }
              }
              frame True {
                n148 = case shown="\"CV\"" w202 {
                  tunnel: [T3."IV" ("Action") T3."CV" ("Action") T3."Reset" ("Action") w212 T3."Interstrip Cap" ("Action") T3."Interstrip Res" ("Action") T3."Reset" ("Action")] -> w201
                  frame "IV", Default {
                  }
                  frame "CV" {
                  }
                  frame "Stability" {
                  }
                  frame "Striptest" {
                    n149 = call <vilib>:"Three Button Dialog.vi"("Allow user to close window? (TRUE)"=TRUE, "Window Title (\"\")"="Select", "Right Button Text (\"Cancel\")"="Ground", "Center Button Text (\"No\")"="RC Test", "Left Button Text (\"Yes\")"="Pinhole Test", "message"="Select striptest settings to test!") -> ("Which Button?"=w214:T11)  [unwired: 5 in]
                    n150 = case shown="\"Left Button\", Default" w214 {
                      tunnel: [T3."Striptest SMU" ("Action") T3."Striptest LCR" ("Action") T3."Ground" ("Action")] -> w212
                      frame "Left Button", Default {
                      }
                      frame "Center Button" {
                      }
                      frame "Right Button" {
                      }
                    }
                  }
                  frame "Cis" {
                  }
                  frame "Ris" {
                  }
                  frame "PTP" {
                  }
                }
                n151 = stacked-sequence {
                  seq-local: [w226 _] -> [_ w229]
                  seq-local: [w225 _] -> [_ w228]
                  tunnel: refnum<class "Switching.lvclass"> refnum ("Switching in") -> [w224 _]
                  tunnel: w201 -> [_ w227]
                  tunnel: w200 -> [w223 _]
                  frame #0 {
                    n152 = To Variant(anything="") -> (Variant=w221:variant)
                    n153 = call-dynamic "Instr_InitObject.vi"("Instrument Configuration"=w221, "Instrument address"=w223, "Switching in"=w224) -> ("error out"=w225:errorcluster, "Switching out"=w226:refnum<class "Switching.lvclass">)  [unwired: 7 in]
                  }
                  frame #1 {
                    n154 = call-dynamic "MatrixSwitch.vi"("error in (no error)"=w228, "Action"=w227, "Switching in"=w229) -> ()  [unwired: 6 in, 3 out]
                  }
                }
              }
            }
          }
          frame 3 {
            n155 = case shown="\"CV\"" w231 {
              tunnel: [w232 w248 w280 w299 w347 w379 w403] -> w230
              frame "IV", Default {
                n156 = flat-sequence {
                  tunnel: [w242] -> w232
                  frame #0 {
                    n157 = Initialize Array(FALSE, 12, 4) -> (w234:bool[][])
                    n158 = local write "Display Matrix"(w234) -> ()
                  }
                  frame #1 {
                    w244 = TRUE
                    n159 = global read "InstrumentSetup.vi" "Pickering MUX & Matrix Configurations"() -> (w241:T4)
                    n160 = Unbundle By Name(w241) -> ("Matrix X Channels.Bias Supply / SMU LO"=w240:i32, "Matrix X Channels.Bias Supply / SMU HI"=w239:i32)
                    n161 = local read "Display Matrix"() -> (w243:bool[][])
                    n162 = Decrement(x=w240) -> (x-1=w237:i32)
                    n163 = Decrement(x=w239) -> (x-1=w238:i32)
                    n164 = Replace Array Subset(array=w243, new element=w244, index (row)=w237, index (col)=1) -> (w245:bool[][])
                    n165 = Replace Array Subset(array=w245, new element=w244, index (row)=w238, index (col)=0) -> (w242:bool[][])
                  }
                }
              }
              frame "CV" {
                n166 = flat-sequence {
                  tunnel: [w266] -> w248
                  frame #0 {
                    n167 = Initialize Array(FALSE, 12, 4) -> (w250:bool[][])
                    n168 = local write "Display Matrix"(w250) -> ()
                  }
                  frame #1 {
                    w268 = TRUE
                    n169 = global read "InstrumentSetup.vi" "Pickering MUX & Matrix Configurations"() -> (w265:T4)
                    n170 = Unbundle By Name(w265) -> ("Matrix X Channels.CV Box LO"=w264:i32, "Matrix X Channels.CV Box HI"=w259:i32, "Matrix X Channels.Bias Supply / SMU LO"=w260:i32, "Matrix X Channels.Bias Supply / SMU HI"=w261:i32, "Matrix X Channels.CV Box LO IN"=w262:i32, "Matrix X Channels.CV Box HI IN"=w263:i32)
                    n171 = local read "Display Matrix"() -> (w267:bool[][])
                    n172 = Decrement(x=w264) -> (x-1=w258:i32)
                    n173 = Decrement(x=w259) -> (x-1=w257:i32)
                    n174 = Decrement(x=w260) -> (x-1=w256:i32)
                    n175 = Decrement(x=w261) -> (x-1=w255:i32)
                    n176 = Decrement(x=w262) -> (x-1=w254:i32)
                    n177 = Decrement(x=w263) -> (x-1=w253:i32)
                    n178 = Replace Array Subset(array=w267, new element=w268, index (row)=w258, index (col)=1) -> (w277:bool[][])
                    n179 = Replace Array Subset(array=w277, new element=w268, index (row)=w257, index (col)=0) -> (w276:bool[][])
                    n180 = Replace Array Subset(array=w276, new element=w268, index (row)=w256, index (col)=2 ("Index")) -> (w275:bool[][])
                    n181 = Replace Array Subset(array=w275, new element=w268, index (row)=w255, index (col)=3 ("Index")) -> (w269:bool[][])
                    n182 = Replace Array Subset(array=w269, new element=w268, index (row)=w254, index (col)=2) -> (w270:bool[][])
                    n183 = Replace Array Subset(array=w270, new element=w268, index (row)=w253, index (col)=3) -> (w266:bool[][])
                  }
                }
              }
              frame "Stability" {
                n184 = flat-sequence {
                  tunnel: [w285] -> w280
                  frame #0 {
                    n185 = Initialize Array(FALSE, 12, 4) -> (w282:bool[][])
                    n186 = local write "Display Matrix"(w282) -> ()
                  }
                  frame #1 {
                    w286 = TRUE
                    n187 = local read "Display Matrix"() -> (w298:bool[][])
                    n188 = Replace Array Subset(array=w298, new element=w286, index (row)=0, index (col)=0) -> (w295:bool[][])
                    n189 = Replace Array Subset(array=w295, new element=w286, index (row)=1, index (col)=1) -> (w288:bool[][])
                    n190 = Replace Array Subset(array=w288, new element=w286, index (row)=2, index (col)=1) -> (w287:bool[][])
                    n191 = Replace Array Subset(array=w287, new element=w286, index (row)=11, index (col)=1) -> (w285:bool[][])
                  }
                }
              }
              frame "Striptest" {
                n192 = flat-sequence {
                  tunnel: [w325] -> w299
                  frame #0 {
                    n193 = Initialize Array(FALSE, 12, 4) -> (w301:bool[][])
                    n194 = local write "Display Matrix"(w301) -> ()
                  }
                  frame #1 {
                    w327 = TRUE
                    n195 = global read "InstrumentSetup.vi" "Pickering MUX & Matrix Configurations"() -> (w324:T4)
                    n196 = Unbundle By Name(w324) -> ("Matrix X Channels.Bias Supply / SMU LO"=w323:i32, "Matrix X Channels.Bias Supply / SMU HI"=w318:i32, "Matrix X Channels.CV Box LO IN"=w319:i32, "Matrix X Channels.CV Box HI IN"=w320:i32, "Matrix X Channels.CV Box LO"=w321:i32, "Matrix X Channels.CV Box HI"=w322:i32, "Matrix X Channels.Mux1 C1"=w314:i32, "Matrix X Channels.Mux1 C2"=w315:i32, "Matrix X Channels.Mux2 C1"=w316:i32, "Matrix X Channels.Mux2 C2"=w317:i32)
                    n197 = local read "Display Matrix"() -> (w335:bool[][])
                    n198 = Decrement(x=w323) -> (x-1=w313:i32)
                    n199 = Decrement(x=w318) -> (x-1=w312:i32)
                    n200 = Decrement(x=w319) -> (x-1=w311:i32)
                    n201 = Decrement(x=w320) -> (x-1=w310:i32)
                    n202 = Decrement(x=w321) -> (x-1=w309:i32)
                    n203 = Decrement(x=w322) -> (x-1=w308:i32)
                    n204 = Decrement(x=w314) -> (x-1=w307:i32)
                    n205 = Decrement(x=w315) -> (x-1=w306:i32)
                    n206 = Decrement(x=w316) -> (x-1=w305:i32)
                    n207 = Decrement(x=w317) -> (x-1=w304:i32)
                    n208 = Replace Array Subset(array=w335, new element=w327, index (row)=w313, index (col)=1) -> (w344:bool[][])
                    n209 = Replace Array Subset(array=w344, new element=w327, index (row)=w312, index (col)=0) -> (w343:bool[][])
                    n210 = Replace Array Subset(array=w343, new element=w327, index (row)=w311, index (col)=3 ("Index")) -> (w342:bool[][])
                    n211 = Replace Array Subset(array=w342, new element=w327, index (row)=w310, index (col)=3 ("Index")) -> (w336:bool[][])
                    n212 = Replace Array Subset(array=w336, new element=w327, index (row)=w309, index (col)=0) -> (w337:bool[][])
                    n213 = Replace Array Subset(array=w337, new element=w327, index (row)=w308, index (col)=1) -> (w326:bool[][])
                    n214 = Replace Array Subset(array=w326, new element=w327, index (row)=w307, index (col)=0) -> (w330:bool[][])
                    n215 = Replace Array Subset(array=w330, new element=w327, index (row)=w306, index (col)=0) -> (w329:bool[][])
                    n216 = Replace Array Subset(array=w329, new element=w327, index (row)=w305, index (col)=0) -> (w328:bool[][])
                    n217 = Replace Array Subset(array=w328, new element=w327, index (row)=w304, index (col)=0) -> (w325:bool[][])
                  }
                }
              }
              frame "Cis" {
                n218 = flat-sequence {
                  tunnel: [w352] -> w347
                  frame #0 {
                    n219 = Initialize Array(FALSE, 12, 4) -> (w349:bool[][])
                    n220 = local write "Display Matrix"(w349) -> ()
                  }
                  frame #1 {
                    w368 = TRUE
                    n221 = global read "InstrumentSetup.vi" "Pickering MUX & Matrix Configurations"() -> (w367:T4)
                    n222 = Unbundle By Name(w367) -> ("Matrix X Channels.CV Box LO"=w366:i32, "Matrix X Channels.CV Box HI"=w361:i32, "Matrix X Channels.Bias Supply / SMU LO"=w362:i32, "Matrix X Channels.Bias Supply / SMU HI"=w363:i32, "Matrix X Channels.CV Box LO IN"=w364:i32, "Matrix X Channels.CV Box HI IN"=w365:i32)
                    n223 = local read "Display Matrix"() -> (w358:bool[][])
                    n224 = Decrement(x=w366) -> (x-1=w360:i32)
                    n225 = Decrement(x=w361) -> (x-1=w359:i32)
                    n226 = Decrement(x=w362) -> (x-1=w356:i32)
                    n227 = Decrement(x=w363) -> (x-1=w355:i32)
                    n228 = Decrement(x=w364) -> (x-1=w354:i32)
                    n229 = Decrement(x=w365) -> (x-1=w353:i32)
                    n230 = Replace Array Subset(array=w358, new element=w368, index (row)=w360, index (col)=2) -> (w369:bool[][])
                    n231 = Replace Array Subset(array=w369, new element=w368, index (row)=w359, index (col)=3) -> (w357:bool[][])
                    n232 = Replace Array Subset(array=w357, new element=w368, index (row)=w356, index (col)=1) -> (w376:bool[][])
                    n233 = Replace Array Subset(array=w376, new element=w368, index (row)=w355, index (col)=0) -> (w375:bool[][])
                    n234 = Replace Array Subset(array=w375, new element=w368, index (row)=w354, index (col)=2 ("Index")) -> (w374:bool[][])
                    n235 = Replace Array Subset(array=w374, new element=w368, index (row)=w353, index (col)=2 ("Index")) -> (w352:bool[][])
                  }
                }
              }
              frame "Ris" {
                n236 = flat-sequence {
                  tunnel: [w393] -> w379
                  frame #0 {
                    n237 = Initialize Array(FALSE, 12, 4) -> (w381:bool[][])
                    n238 = local write "Display Matrix"(w381) -> ()
                  }
                  frame #1 {
                    w394 = TRUE
                    n239 = global read "InstrumentSetup.vi" "Pickering MUX & Matrix Configurations"() -> (w392:T4)
                    n240 = Unbundle By Name(w392) -> ("Matrix X Channels.Volt meter LO"=w391:i32, "Matrix X Channels.Volt meter HI"=w388:i32, "Matrix X Channels.Bias Supply / SMU LO"=w389:i32, "Matrix X Channels.Bias Supply / SMU HI"=w390:i32)
                    n241 = local read "Display Matrix"() -> (w402:bool[][])
                    n242 = Decrement(x=w391) -> (x-1=w384:i32)
                    n243 = Decrement(x=w388) -> (x-1=w385:i32)
                    n244 = Decrement(x=w389) -> (x-1=w387:i32)
                    n245 = Decrement(x=w390) -> (x-1=w386:i32)
                    n246 = Replace Array Subset(array=w402, new element=w394, index (row)=w384, index (col)=1) -> (w400:bool[][])
                    n247 = Replace Array Subset(array=w400, new element=w394, index (row)=w385, index (col)=3) -> (w397:bool[][])
                    n248 = Replace Array Subset(array=w397, new element=w394, index (row)=w387, index (col)=1) -> (w395:bool[][])
                    n249 = Replace Array Subset(array=w395, new element=w394, index (row)=w386, index (col)=2) -> (w393:bool[][])
                  }
                }
              }
              frame "PTP" {
                n250 = flat-sequence {
                  tunnel: [w405] -> w404
                  tunnel: w404 -> [w409]
                  tunnel: [w409] -> w403
                  frame #0 {
                    n251 = Initialize Array(FALSE, 12, 4) -> (w405:bool[][])
                    n252 = local write "Display Matrix"(w405) -> ()
                  }
                  frame #1 {
                  }
                }
              }
            }
            n253 = local write "Display Matrix"(w230) -> ()
          }
        }
        n254 = Not(x="No Matrix") -> (.not. x?=w149:bool)
        n255 = Number To Decimal String(number="Matrix address") -> (decimal integer string=w164:string)  [unwired: 1 in]
        n256 = Number To Decimal String(number="Mux1 address") -> (decimal integer string=w162:string)  [unwired: 1 in]
        n257 = Number To Decimal String(number="Mux2 address") -> (decimal integer string=w163:string)  [unwired: 1 in]
        n258 = Bundle By Name(cluster=w157, "Matrix address"=w164, "Mux1 address"=w162, "Mux2 address"=w163, "Matrix used?"=w149) -> (w156:T4)
        n259 = case shown="\"WayneKerr 6425\"" "LCRs" {
          tunnel: "Defaults LCR" -> [w431 w451]
          tunnel: w128 -> [w428 w449]
          tunnel: [w426 w448] -> w131
          frame "WayneKerr 6440B", Default {
            n260 = case shown="True" w431 {
              tunnel: w428 -> [_ w443]
              frame False {
              }
              frame True {
                n261 = Unbundle By Name(w443) -> ("WK 6440B.GPIB address"=w442)
                n262 = local write "AC amplitude [V]"(0.1) -> ()
                n263 = global read "QC_RunInformation.vi" "Run info"() -> (w437:T12)
                n264 = Decimal String To Number(string=w442) -> (number=w441:i32)  [unwired: 2 in, 1 out]
                n265 = local write "GPIB Address WK6440B"(w441) -> ()
                n266 = Unbundle By Name(w437) -> ("Test"=w436:string)
                n267 = case shown="\"CV\", Default" w436 {
                  tunnel: [w445 w447] -> w439
                  tunnel: [100000 1000] -> w438
                  frame "Cis" {
                    w445 = u16 1 items=["serial", "parallel"] ("RC Configuration")
                  }
                  frame "CV", Default {
                    w447 = u16 0 items=["serial", "parallel"] ("RC Configuration")
                  }
                }
                n268 = local write "RC Configuration"(w439) -> ()
                n269 = local write "AC frequency [Hz]"(w438) -> ()
              }
            }
            n270 = global read "InstrumentSetup.vi" "WayneKerr 6440B Configurations"() -> (w435:T13)
            n271 = Bundle By Name(cluster=w435, "RC Configuration"="RC Configuration", "AC amplitude [V]"="AC amplitude [V]", "AC frequency [Hz]"="AC frequency [Hz]") -> (w434:T13)
            n272 = global write "InstrumentSetup.vi" "WayneKerr 6440B Configurations"(w434) -> ()
            n273 = Number To Decimal String(number="GPIB Address WK6440B") -> (decimal integer string=w427:string)  [unwired: 1 in]
            n274 = Bundle By Name(cluster=w428, "GPIB address"=w427) -> (w426:cluster{})
          }
          frame "WayneKerr 6425" {
            n275 = case shown="True" w451 {
              tunnel: w449 -> [_ w465]
              frame False {
              }
              frame True {
                n276 = Unbundle By Name(w465) -> ("WK 6425.GPIB address"=w464)
                n277 = local write "AC amplitude [V] WK6425"(0.1) -> ()
                n278 = global read "QC_RunInformation.vi" "Run info"() -> (w459:T12)
                n279 = Decimal String To Number(string=w464) -> (number=w463:i32)  [unwired: 2 in, 1 out]
                n280 = local write "GPIB Address WK6425"(w463) -> ()
                n281 = Unbundle By Name(w459) -> ("Test"=w458:string)
                n282 = case shown="\"CV\", Default" w458 {
                  tunnel: [w467 w469] -> w461
                  tunnel: [100000 1000] -> w460
                  frame "Cis" {
                    w467 = u16 1 items=["serial", "parallel"] ("RC Configuration")
                  }
                  frame "CV", Default {
                    w469 = u16 0 items=["serial", "parallel"] ("RC Configuration")
                  }
                }
                n283 = local write "RC Configuration WK6425"(w461) -> ()
                n284 = local write "AC frequency [Hz] WK6425"(w460) -> ()
              }
            }
            n285 = global read "InstrumentSetup.vi" "WayneKerr 6425 Configurations"() -> (w453:T14)
            n286 = Bundle By Name(cluster=w453, "RC Configuration"="RC Configuration WK6425", "AC amplitude [V]"="AC amplitude [V] WK6425", "AC frequency [Hz]"="AC frequency [Hz] WK6425") -> (w452:T14)
            n287 = global write "InstrumentSetup.vi" "WayneKerr 6425 Configurations"(w452) -> ()
            n288 = Number To Decimal String(number="GPIB Address WK6425") -> (decimal integer string=w450:string)  [unwired: 1 in]
            n289 = Bundle By Name(cluster=w449, "GPIB address"=w450) -> (w448:cluster{})
          }
        }
        n290 = case shown="\"Keithley 236\"" "Supplies" {
          tunnel: "Defaults Supply" -> [w810 w823 w836 w849]
          tunnel: w128 -> [w801 w816 w831 w842]
          tunnel: [w802 w815 w830 w843] -> w130
          frame "Keithley 2410", Default {
            n291 = case shown="True" w810 {
              tunnel: w801 -> [_ w814]
              frame False {
              }
              frame True {
                n292 = Unbundle By Name(w814) -> ("KE 2410.GPIB address"=w813)
                n293 = local write "Current Limit [µA]"(100.0) -> ()
                n294 = Decimal String To Number(string=w813) -> (number=w812:i32)  [unwired: 2 in, 1 out]
                n295 = local write "GPIB Address KE2410"(w812) -> ()
              }
            }
            n296 = global read "InstrumentSetup.vi" "Keithley 2410 Configurations"() -> (w809:T15)
            n297 = Divide(x="Current Limit [µA]", y=1000000.0) -> (x/y=w804:dbl)
            n298 = Bundle By Name(cluster=w809, "Current Limit"=w804) -> (w808:T15)
            n299 = global write "InstrumentSetup.vi" "Keithley 2410 Configurations"(w808) -> ()
            n300 = Number To Decimal String(number="GPIB Address KE2410") -> (decimal integer string=w803:string)  [unwired: 1 in]
            n301 = Bundle By Name(cluster=w801, "GPIB address"=w803) -> (w802:cluster{})
          }
          frame "Keithley 487" {
            n302 = case shown="True" w823 {
              tunnel: w816 -> [_ w828]
              frame False {
              }
              frame True {
                w824 = u16 0 items=["Autorange", "2nA", "20nA", "200nA", "2 microAmp", "20 microAmp", "200 microAmp", "2 milliAmp"] ("Range:")
                w825 = u16 0 items=["20µA", "2mA"] ("Compliance")
                n303 = Unbundle By Name(w828) -> ("KE 487.GPIB address"=w827)
                n304 = local write "Compliance"(w825) -> ()
                n305 = Decimal String To Number(string=w827) -> (number=w826:i32)  [unwired: 2 in, 1 out]
                n306 = local write "GPIB Address KE487"(w826) -> ()
                n307 = local write "Range:"(w824) -> ()
              }
            }
            n308 = global read "InstrumentSetup.vi" "Keithley 487 Configurations"() -> (w822:T16)
            n309 = Bundle By Name(cluster=w822, "Compliance"="Compliance", "Range:"="Range:") -> (w821:T16)
            n310 = global write "InstrumentSetup.vi" "Keithley 487 Configurations"(w821) -> ()
            n311 = Number To Decimal String(number="GPIB Address KE487") -> (decimal integer string=w817:string)  [unwired: 1 in]
            n312 = Bundle By Name(cluster=w816, "GPIB address"=w817) -> (w815:cluster{})
          }
          frame "Keithley 6517" {
            n313 = case shown="True" w836 {
              tunnel: w831 -> [_ w840]
              frame False {
              }
              frame True {
                w837 = u16 1 items=["OFF", "ON"] ("Current Limit")
                n314 = Unbundle By Name(w840) -> ("KE 6517.GPIB address"=w838)
                n315 = local write "Current Limit"(w837) -> ()
                n316 = Decimal String To Number(string=w838) -> (number=w839:i32)  [unwired: 2 in, 1 out]
                n317 = local write "GPIB Address KE6517"(w839) -> ()
              }
            }
            n318 = global read "InstrumentSetup.vi" "Keithley 6517 Configurations"() -> (w835:T17)
            n319 = Bundle By Name(cluster=w835, "Current Limit"="Current Limit") -> (w834:T17)
            n320 = global write "InstrumentSetup.vi" "Keithley 6517 Configurations"(w834) -> ()
            n321 = Number To Decimal String(number="GPIB Address KE6517") -> (decimal integer string=w829:string)  [unwired: 1 in]
            n322 = Bundle By Name(cluster=w831, "GPIB address"=w829) -> (w830:cluster{})
          }
          frame "Keithley 236" {
            n323 = case shown="True" w849 {
              tunnel: w842 -> [_ w854]
              frame False {
              }
              frame True {
                w850 = u16 6 items=["auto / auto", "1 nA / 1.1 V", "10 nA / 11 V", "100 nA / 110 V", "0.001 mA / 110 V", "0.01 mA / 110 V", "0.1 mA / 110 V", "1 mA / 110 V", "10 mA / 110 V", "100 mA / 110 V"] ("compliance/\nmeasurement range (auto:0)")
                n324 = Unbundle By Name(w854) -> ("KE 236.GPIB address"=w853)
                n325 = local write "current compliance \nlevel [mA]"(0.0001 ("current \ncompliance level")) -> ()
                n326 = Decimal String To Number(string=w853) -> (number=w852:i32)  [unwired: 2 in, 1 out]
                n327 = local write "GPIB Address KE236"(w852) -> ()
                n328 = local write "compliance/\nmeasurement range (auto:0)"(w850) -> ()
              }
            }
            n329 = global read "InstrumentSetup.vi" "Keithley 236 Configurations"() -> (w845:T18)
            n330 = Bundle By Name(cluster=w845, "current \ncompliance level"="current compliance \nlevel [mA]", "compliance/\nmeasurement range (auto:0)"="compliance/\nmeasurement range (auto:0)") -> (w846:T18)
            n331 = global write "InstrumentSetup.vi" "Keithley 236 Configurations"(w846) -> ()
            n332 = Number To Decimal String(number="GPIB Address KE236") -> (decimal integer string=w841:string)  [unwired: 1 in]
            n333 = Bundle By Name(cluster=w842, "GPIB address"=w841) -> (w843:cluster{})
          }
        }
        n334 = global write "InstrumentSetup.vi" "Instrument GPIB addresses"(w127) -> ()
        n335 = global write "InstrumentSetup.vi" "Pickering MUX & Matrix Configurations"(w156) -> ()
        n336 = local write "Change Preset Parameters"(w166) -> ()
        n337 = case shown="\"Striptest\"" "Measurements" {
          tunnel: w166 -> [w516 w573 w611 w648 w707 w757 _]
          frame "IV", Default {
            w480 = "" ("Input Element")
            w511 = ""
            n338 = Select(t=0, s=w516, f=2) -> (s? t:f=w514:i32)
            n339 = property on="V_breakdown Limit [V]" class="DigNum (strict)"("DisabledEnum"=w514) -> ()  [unwired: 2 in, 2 out]
            n340 = property on="IV Ramp down Interval [s]" class="DigNum (strict)"("DisabledEnum"=w514) -> ()  [unwired: 2 in, 2 out]
            n341 = property on="IV Step Size [V]" class="DigNum (strict)"("DisabledEnum"=w514) -> ()  [unwired: 2 in, 2 out]
            n342 = property on="IV Ramp down steps [V]" class="DigNum (strict)"("DisabledEnum"=w514) -> ()  [unwired: 2 in, 2 out]
            n343 = property on="IV Final Voltage [V]" class="DigNum (strict)"("DisabledEnum"=w514) -> ()  [unwired: 2 in, 2 out]
            n344 = property on="IV Initial Voltage [V]" class="DigNum (strict)"("DisabledEnum"=w514) -> ()  [unwired: 2 in, 2 out]
            n345 = property on="IV Step Interval [s]" class="DigNum (strict)"("DisabledEnum"=w514) -> ()  [unwired: 2 in, 2 out]
            n346 = local read "Y Mapping"() -> (w505:string[])
            n347 = case shown="True" "Save IV defaults" {
              frame False {
              }
              frame True {
              }
            }
            n348 = Replace Array Subset(array=w505, new element #1="Backplane" ("String"), index #1=0, new element #2="Bias Rail (GND)" ("String"), index #2=1, new element #3=w511, index #3=2, new element #4=w511, index #4=3) -> (w506:string[])
            n349 = Absolute Value(x="IV Final Voltage [V]") -> (abs(x)=w523:dbl)
            n350 = Absolute Value(x="IV Initial Voltage [V]") -> (abs(x)=w522:dbl)
            n351 = local write "Y Mapping"(w506) -> ()
            n352 = Subtract(x=w523, y=w522) -> (x-y=w521:dbl)
            n353 = global read "InstrumentSetup.vi" "Pickering MUX & Matrix Configurations"() -> (w491:T4)
            n354 = Absolute Value(x=w521) -> (abs(x)=w520:dbl)
            n355 = Absolute Value(x="IV Step Size [V]") -> (abs(x)=w526:dbl)
            n356 = Quotient & Remainder(x=w520, y=w526) -> (floor(x/y)=w518:dbl)  [unwired: 1 out]
            n357 = Unbundle By Name(w491) -> ("Matrix X Channels.CV Box LO"=w485:i32, "Matrix X Channels.CV Box HI"=w486:i32, "Matrix X Channels.CV Box LO IN"=w487:i32, "Matrix X Channels.CV Box HI IN"=w484:i32, "Matrix X Channels.Volt meter LO"=w489:i32, "Matrix X Channels.Volt meter HI"=w488:i32, "Matrix X Channels.Mux1 C1"=w495:i32, "Matrix X Channels.Mux1 C2"=w496:i32, "Matrix X Channels.Mux2 C1"=w493:i32, "Matrix X Channels.Mux2 C2"=w494:i32)
            n358 = global read "QC_MeasurementSetup.vi" "IV Measurement Parameters"() -> (w534:T8)
            n359 = Increment(x=w518) -> (x+1=w517:dbl)
            n360 = call "InstrumentSelection.vi"("Verify GPIB address"=FALSE, "Instrument type"=enum16{"Supply", "LCR", "Multimeter"}."Supply", "Instrument name IN"="IV Voltage Supply") -> ("Instrument name OUT"=w529:string, "Supply"=w530:refnum<class "SupplyControl.lvclass">)  [unwired: 3 in, 4 out]
            n361 = local read "X Mapping CB Standard"() -> (w492:string[])
            n362 = Bundle By Name(cluster=w534, "Supply"=w530, "Initial Voltage [V]"="IV Initial Voltage [V]", "Final Voltage [V]"="IV Final Voltage [V]", "Step Size [V]"="IV Step Size [V]", "Step Interval [s]"="IV Step Interval [s]", "Number Of Steps"=w517, "Ramp down steps [V]"="IV Ramp down steps [V]", "Ramp down Interval [s]"="IV Ramp down Interval [s]", "Temperature Readout"="IV Temperature Readout", "Supply Name"=w529, "V_breakdown Limit [V]"="V_breakdown Limit [V]") -> (w535:T8)
            n363 = Decrement(x=w485) -> (x-1=w479:i32)
            n364 = Decrement(x=w486) -> (x-1=w481:i32)
            n365 = Decrement(x=w487) -> (x-1=w482:i32)
            n366 = Decrement(x=w484) -> (x-1=w483:i32)
            n367 = Decrement(x=w489) -> (x-1=w497:i32)
            n368 = Decrement(x=w488) -> (x-1=w498:i32)
            n369 = Decrement(x=w495) -> (x-1=w499:i32)
            n370 = Decrement(x=w496) -> (x-1=w500:i32)
            n371 = Decrement(x=w493) -> (x-1=w501:i32)
            n372 = Decrement(x=w494) -> (x-1=w502:i32)
            n373 = global write "QC_MeasurementSetup.vi" "IV Measurement Parameters"(w535) -> ()
            n374 = Replace Array Subset(array=w492, new element #1=w480, index #1=w479, new element #2=w480, index #2=w481, new element #3=w480, index #3=w482, new element #4=w480, index #4=w483, new element #5=w480, index #5=w497, new element #6=w480, index #6=w498, new element #7=w480, index #7=w499, new element #8=w480, index #8=w500, new element #9=w480, index #9=w501, new element #10=w480, index #10=w502) -> (w490:string[])
            n375 = local write "X Mapping"(w490) -> ()
          }
          frame "CV" {
            w538 = FALSE
            w548 = "" ("Input Element")
            w563 = ""
            w568 = u16 0 items=["serial", "parallel"] ("RC Configuration")
            n376 = Select(t=0, s=w573, f=2) -> (s? t:f=w566:i32)
            n377 = property on="V_depletion Limit [V]" class="DigNum (strict)"("DisabledEnum"=w566) -> ()  [unwired: 2 in, 2 out]
            n378 = property on="CV Ramp down steps [V]" class="DigNum (strict)"("DisabledEnum"=w566) -> ()  [unwired: 2 in, 2 out]
            n379 = property on="CV Final Voltage [V]" class="DigNum (strict)"("DisabledEnum"=w566) -> ()  [unwired: 2 in, 2 out]
            n380 = property on="CV Ramp down Interval [s]" class="DigNum (strict)"("DisabledEnum"=w566) -> ()  [unwired: 2 in, 2 out]
            n381 = property on="CV Initial Voltage [V]" class="DigNum (strict)"("DisabledEnum"=w566) -> ()  [unwired: 2 in, 2 out]
            n382 = property on="CV Step Size [V]" class="DigNum (strict)"("DisabledEnum"=w566) -> ()  [unwired: 2 in, 2 out]
            n383 = property on="CV Step Interval [s]" class="DigNum (strict)"("DisabledEnum"=w566) -> ()  [unwired: 2 in, 2 out]
            n384 = local read "Y Mapping"() -> (w557:string[])
            n385 = case shown="True" "Save CV defaults" {
              frame False {
              }
              frame True {
              }
            }
            n386 = Replace Array Subset(array=w557, new element #1="Backplane" ("String"), index #1=0, new element #2="Bias Rail (GND)" ("String"), index #2=1, new element #3=w563, index #3=2, new element #4=w563, index #4=3) -> (w558:string[])
            n387 = Absolute Value(x="CV Final Voltage [V]") -> (abs(x)=w588:dbl)
            n388 = Absolute Value(x="CV Initial Voltage [V]") -> (abs(x)=w587:dbl)
            n389 = local write "Y Mapping"(w558) -> ()
            n390 = Subtract(x=w588, y=w587) -> (x-y=w586:dbl)
            n391 = global read "InstrumentSetup.vi" "Pickering MUX & Matrix Configurations"() -> (w542:T4)
            n392 = Absolute Value(x=w586) -> (abs(x)=w585:dbl)
            n393 = Absolute Value(x="CV Step Size [V]") -> (abs(x)=w589:dbl)
            n394 = call "InstrumentSelection.vi"("Verify GPIB address"=w538, "Instrument type"=enum16{"Supply", "LCR", "Multimeter"}."Supply", "Instrument name IN"="CV Voltage Supply") -> ("error out"=w571:errorcluster, "Instrument name OUT"=w579:string, "Supply"=w577:refnum<class "SupplyControl.lvclass">)  [unwired: 3 in, 3 out]
            n395 = Quotient & Remainder(x=w585, y=w589) -> (floor(x/y)=w584:dbl)  [unwired: 1 out]
            n396 = Unbundle By Name(w542) -> ("Matrix X Channels.Volt meter LO"=w540:i32, "Matrix X Channels.Volt meter HI"=w539:i32, "Matrix X Channels.Mux1 C1"=w546:i32, "Matrix X Channels.Mux1 C2"=w547:i32, "Matrix X Channels.Mux2 C1"=w544:i32, "Matrix X Channels.Mux2 C2"=w545:i32)
            n397 = global read "QC_MeasurementSetup.vi" "CV Measurement Parameters"() -> (w594:T6)
            n398 = call "InstrumentSelection.vi"("error in (no error)"=w571, "Verify GPIB address"=w538, "Instrument type"=enum16{"Supply", "LCR", "Multimeter"}."LCR", "Instrument name IN"="CV LCR Meter") -> ("Instrument name OUT"=w569:string, "LCR"=w570:refnum<class "LCRControl.lvclass">)  [unwired: 2 in, 4 out]
            n399 = Increment(x=w584) -> (x+1=w580:dbl)
            n400 = local read "X Mapping CB Standard"() -> (w543:string[])
            n401 = Decrement(x=w540) -> (x-1=w549:i32)
            n402 = Decrement(x=w539) -> (x-1=w550:i32)
            n403 = Decrement(x=w546) -> (x-1=w551:i32)
            n404 = Decrement(x=w547) -> (x-1=w552:i32)
            n405 = Decrement(x=w544) -> (x-1=w553:i32)
            n406 = Decrement(x=w545) -> (x-1=w554:i32)
            n407 = Bundle By Name(cluster=w594, "Supply"=w577, "LCR"=w570, "Initial Voltage [V]"="CV Initial Voltage [V]", "Final Voltage [V]"="CV Final Voltage [V]", "Step Size [V]"="CV Step Size [V]", "Step Interval [s]"="CV Step Interval [s]", "Number Of Steps"=w580, "RC Configuration"=w568, "Ramp down steps [V]"="CV Ramp down steps [V]", "Ramp down Interval [s]"="CV Ramp down Interval [s]", "Temperature Readout"="CV Temperature Readout", "Supply Name"=w579, "LCR Name"=w569, "V_depletion Limit [V]"="V_depletion Limit [V]") -> (w595:T6)
            n408 = global write "QC_MeasurementSetup.vi" "CV Measurement Parameters"(w595) -> ()
            n409 = Replace Array Subset(array=w543, new element #1=w548, index #1=w549, new element #2=w548, index #2=w550, new element #3=w548, index #3=w551, new element #4=w548, index #4=w552, new element #5=w548, index #5=w553, new element #6=w548, index #6=w554) -> (w541:string[])
            n410 = local write "X Mapping"(w541) -> ()
          }
          frame "Stability" {
            w599 = 11
            w607 = ""
            n411 = Select(t=0, s=w611, f=2) -> (s? t:f=w610:i32)
            n412 = property on="Maximum current fluctuation [%]" class="DigNum (strict)"("DisabledEnum"=w610) -> ()  [unwired: 2 in, 2 out]
            n413 = local read "Y Mapping"() -> (w602:string[])
            n414 = local read "X Mapping CB Standard"() -> (w600:string[])
            n415 = Replace Array Subset(array=w602, new element #1="Amp meter HI" ("String"), index #1=0, new element #2="Bias Supply LO" ("String"), index #2=1, new element #3=w607, index #3=2, new element #4=w607, index #4=3) -> (w603:string[])
            n416 = for {
              N: w599 -> [_]
              shift-right: [w620] -> w597
              shift-left: w600 -> [w621]
              i -> [w622]
              n417 = Increment(x=w622) -> (x+1=w618:i32)
              n418 = Format Into String(format string="Sensor %d", w618) -> (resulting string=w615:string)  [unwired: 2 in, 1 out]
              n419 = Less Or Equal?(x=w618, y=3) -> (x <= y?=w619:bool)
              n420 = Select(t=w615, s=w619, f="     ...     ") -> (s? t:f=w614:string)
              n421 = Replace Array Subset(array=w621, new element=w614, index=w622) -> (w620:string[])
            }
            n422 = local write "Y Mapping"(w603) -> ()
            n423 = Replace Array Subset(array=w597, new element="Amp meter LO", index=w599) -> (w596:string[])
            n424 = local write "X Mapping"(w596) -> ()
          }
          frame "Striptest" {
            w626 = "" ("Input Element")
            w646 = ""
            n425 = Select(t=0, s=w648, f=2) -> (s? t:f=w647:i32)
            n426 = property on="Fraction of good strips [%]" class="DigNum (strict)"("DisabledEnum"=w647) -> ()  [unwired: 2 in, 2 out]
            n427 = local read "Y Mapping"() -> (w640:string[])
            n428 = Replace Array Subset(array=w640, new element #1="Probe Needle(s)" ("String"), index #1=0, new element #2="Common GND" ("String"), index #2=1, new element #3=w646, index #3=2, new element #4=w646, index #4=3) -> (w641:string[])
            n429 = local write "Y Mapping"(w641) -> ()
            n430 = global read "InstrumentSetup.vi" "Pickering MUX & Matrix Configurations"() -> (w636:T4)
            n431 = Unbundle By Name(w636) -> ("Matrix X Channels.Bias Supply / SMU LO"=w635:i32, "Matrix X Channels.Bias Supply / SMU HI"=w634:i32, "Matrix X Channels.Volt meter LO"=w630:i32, "Matrix X Channels.Volt meter HI"=w629:i32)
            n432 = local read "X Mapping CB Standard"() -> (w637:string[])
            n433 = Decrement(x=w635) -> (x-1=w633:i32)
            n434 = Decrement(x=w634) -> (x-1=w631:i32)
            n435 = Decrement(x=w630) -> (x-1=w628:i32)
            n436 = Decrement(x=w629) -> (x-1=w627:i32)
            n437 = Replace Array Subset(array=w637, new element #1="SMU LO (GND)" ("Input Element"), index #1=w633, new element #2="SMU HI" ("Input Element"), index #2=w631, new element #3=w626, index #3=w628, new element #4=w626, index #4=w627) -> (w632:string[])
            n438 = local write "X Mapping"(w632) -> ()
          }
          frame "Cis" {
            w651 = FALSE
            w665 = "" ("Input Element")
            w682 = u16 1 items=["serial", "parallel"] ("RC Configuration")
            n439 = Select(t=0, s=w707, f=2) -> (s? t:f=w681:i32)
            n440 = property on="C_is Limit [pF/cm]" class="DigNum (strict)"("DisabledEnum"=w681) -> ()  [unwired: 2 in, 2 out]
            n441 = property on="Cis Ramp down Interval [s]" class="DigNum (strict)"("DisabledEnum"=w681) -> ()  [unwired: 2 in, 2 out]
            n442 = property on="Cis Initial Voltage [V]" class="DigNum (strict)"("DisabledEnum"=w681) -> ()  [unwired: 2 in, 2 out]
            n443 = property on="Cis Ramp down steps [V]" class="DigNum (strict)"("DisabledEnum"=w681) -> ()  [unwired: 2 in, 2 out]
            n444 = property on="Cis Final Voltage [V]" class="DigNum (strict)"("DisabledEnum"=w681) -> ()  [unwired: 2 in, 2 out]
            n445 = property on="Cis Step Size [V]" class="DigNum (strict)"("DisabledEnum"=w681) -> ()  [unwired: 2 in, 2 out]
            n446 = property on="Cis Step Interval [s]" class="DigNum (strict)"("DisabledEnum"=w681) -> ()  [unwired: 2 in, 2 out]
            n447 = case shown="True" "Save Cis defaults" {
              frame False {
              }
              frame True {
              }
            }
            n448 = local read "Y Mapping"() -> (w673:string[])
            n449 = Absolute Value(x="Cis Final Voltage [V]") -> (abs(x)=w691:dbl)
            n450 = Absolute Value(x="Cis Initial Voltage [V]") -> (abs(x)=w690:dbl)
            n451 = Replace Array Subset(array=w673, new element #1="Backplane" ("String"), index #1=0, new element #2="Bias Rail (GND)" ("String"), index #2=1, new element #3="Neighbour Strips" ("String"), index #3=2, new element #4="Centre Strip" ("String"), index #4=3) -> (w674:string[])
            n452 = Subtract(x=w691, y=w690) -> (x-y=w689:dbl)
            n453 = global read "InstrumentSetup.vi" "Pickering MUX & Matrix Configurations"() -> (w659:T4)
            n454 = local write "Y Mapping"(w674) -> ()
            n455 = Absolute Value(x=w689) -> (abs(x)=w688:dbl)
            n456 = Absolute Value(x="Cis Step Size [V]") -> (abs(x)=w692:dbl)
            n457 = call "InstrumentSelection.vi"("Verify GPIB address"=w651, "Instrument type"=enum16{"Supply", "LCR", "Multimeter"}."Supply", "Instrument name IN"="Cis Voltage Supply") -> ("error out"=w703:errorcluster, "Instrument name OUT"=w699:string, "Supply"=w700:refnum<class "SupplyControl.lvclass">)  [unwired: 3 in, 3 out]
            n458 = Quotient & Remainder(x=w688, y=w692) -> (floor(x/y)=w684:dbl)  [unwired: 1 out]
            n459 = Unbundle By Name(w659) -> ("Matrix X Channels.Volt meter LO"=w657:i32, "Matrix X Channels.Volt meter HI"=w656:i32, "Matrix X Channels.Mux1 C1"=w663:i32, "Matrix X Channels.Mux1 C2"=w664:i32, "Matrix X Channels.Mux2 C1"=w661:i32, "Matrix X Channels.Mux2 C2"=w662:i32)
            n460 = global read "QC_MeasurementSetup.vi" "Cis Measurement Parameters"() -> (w705:T7)
            n461 = call "InstrumentSelection.vi"("error in (no error)"=w703, "Verify GPIB address"=w651, "Instrument type"=enum16{"Supply", "LCR", "Multimeter"}."LCR", "Instrument name IN"="Cis LCR Meter") -> ("Instrument name OUT"=w698:string, "LCR"=w701:refnum<class "LCRControl.lvclass">)  [unwired: 2 in, 4 out]
            n462 = Increment(x=w684) -> (x+1=w683:dbl)
            n463 = local read "X Mapping CB Standard"() -> (w660:string[])
            n464 = Bundle By Name(cluster=w705, "Supply"=w700, "LCR"=w701, "Initial Voltage [V]"="Cis Initial Voltage [V]", "Final Voltage [V]"="Cis Final Voltage [V]", "Step Size [V]"="Cis Step Size [V]", "Step Interval [s]"="Cis Step Interval [s]", "Number Of Steps"=w683, "RC Configuration"=w682, "Ramp down steps [V]"="Cis Ramp down steps [V]", "Ramp down Interval [s]"="Cis Ramp down Interval [s]", "Temperature Readout"="Cis Temperature Readout", "Supply Name"=w699, "LCR Name"=w698, "C_is Limit [pF/cm]"="C_is Limit [pF/cm]") -> (w706:T7)
            n465 = Decrement(x=w657) -> (x-1=w666:i32)
            n466 = Decrement(x=w656) -> (x-1=w667:i32)
            n467 = Decrement(x=w663) -> (x-1=w668:i32)
            n468 = Decrement(x=w664) -> (x-1=w669:i32)
            n469 = Decrement(x=w661) -> (x-1=w670:i32)
            n470 = Decrement(x=w662) -> (x-1=w671:i32)
            n471 = global write "QC_MeasurementSetup.vi" "Cis Measurement Parameters"(w706) -> ()
            n472 = Replace Array Subset(array=w660, new element #1=w665, index #1=w666, new element #2=w665, index #2=w667, new element #3=w665, index #3=w668, new element #4=w665, index #4=w669, new element #5=w665, index #5=w670, new element #6=w665, index #6=w671) -> (w658:string[])
            n473 = local write "X Mapping"(w658) -> ()
          }
          frame "Ris" {
            w720 = FALSE
            w739 = "" ("Input Element")
            w781 = enum16{"Supply", "LCR", "Multimeter"}."Supply" ("Instrument type")
            n474 = Select(t=0, s=w757, f=2) -> (s? t:f=w756:i32)
            n475 = property on="Ris Initial Voltage [V]" class="DigNum (strict)"("DisabledEnum"=w756) -> ()  [unwired: 2 in, 2 out]
            n476 = property on="Ris Ramp down Interval [s]" class="DigNum (strict)"("DisabledEnum"=w756) -> ()  [unwired: 2 in, 2 out]
            n477 = property on="Ris Step Size [V]" class="DigNum (strict)"("DisabledEnum"=w756) -> ()  [unwired: 2 in, 2 out]
            n478 = property on="Ris Step Interval [s]" class="DigNum (strict)"("DisabledEnum"=w756) -> ()  [unwired: 2 in, 2 out]
            n479 = property on="Ris Ramp down steps [V]" class="DigNum (strict)"("DisabledEnum"=w756) -> ()  [unwired: 2 in, 2 out]
            n480 = property on="Ris Final Voltage [V]" class="DigNum (strict)"("DisabledEnum"=w756) -> ()  [unwired: 2 in, 2 out]
            n481 = property on="R_is Limit [MOhm]" class="DigNum (strict)"("DisabledEnum"=w756) -> ()  [unwired: 2 in, 2 out]
            n482 = local read "Y Mapping"() -> (w748:string[])
            n483 = case shown="True" "Save Ris defaults" {
              frame False {
              }
              frame True {
              }
            }
            n484 = local read "Y Mapping"() -> (w715:string[])
            n485 = Absolute Value(x="Ris Final Voltage [V]") -> (abs(x)=w771:dbl)
            n486 = Absolute Value(x="Ris Initial Voltage [V]") -> (abs(x)=w770:dbl)
            n487 = Replace Array Subset(array=w748, new element #1="Centre Strip" ("String"), index #1=0, new element #2="High Strip" ("String"), index #2=1, new element #3="Ground Strip" ("String"), index #3=2, new element #4="", index #4=3) -> ()  [unwired: 1 out]
            n488 = Replace Array Subset(array=w715, new element #1="", index #1=0, new element #2="Common GND" ("String"), index #2=1, new element #3="Neighbour Strip(s)" ("String"), index #3=2, new element #4="Centre Strip" ("String"), index #4=3) -> (w716:string[])
            n489 = Subtract(x=w771, y=w770) -> (x-y=w769:dbl)
            n490 = call "InstrumentSelection.vi"("Verify GPIB address"=w720, "Instrument type"=w781, "Instrument name IN"="Ris Bias Supply") -> ("error out"=w783:errorcluster, "Instrument name OUT"=w777:string, "Supply"=w780:refnum<class "SupplyControl.lvclass">)  [unwired: 3 in, 3 out]
            n491 = global read "InstrumentSetup.vi" "Pickering MUX & Matrix Configurations"() -> (w729:T4)
            n492 = local write "Y Mapping"(w716) -> ()
            n493 = Absolute Value(x="Ris Step Size [V]") -> (abs(x)=w765:dbl)
            n494 = Absolute Value(x=w769) -> (abs(x)=w766:dbl)
            n495 = Quotient & Remainder(x=w766, y=w765) -> (floor(x/y)=w763:dbl)  [unwired: 1 out]
            n496 = call "InstrumentSelection.vi"("error in (no error)"=w783, "Verify GPIB address"=w720, "Instrument type"=w781, "Instrument name IN"="Ris SMU") -> ("error out"=w782:errorcluster, "Instrument name OUT"=w776:string, "Supply"=w779:refnum<class "SupplyControl.lvclass">)  [unwired: 2 in, 3 out]
            n497 = Unbundle By Name(w729) -> ("Matrix X Channels.Bias Supply / SMU LO"=w741:i32, "Matrix X Channels.Bias Supply / SMU HI"=w742:i32, "Matrix X Channels.CV Box LO"=w725:i32, "Matrix X Channels.CV Box HI"=w726:i32, "Matrix X Channels.CV Box LO IN"=w727:i32, "Matrix X Channels.CV Box HI IN"=w724:i32, "Matrix X Channels.Mux1 C1"=w733:i32, "Matrix X Channels.Mux1 C2"=w734:i32, "Matrix X Channels.Mux2 C1"=w731:i32, "Matrix X Channels.Mux2 C2"=w732:i32)
            n498 = global read "QC_MeasurementSetup.vi" "Ris Measurement Parameters"() -> (w789:T5)
            n499 = call "InstrumentSelection.vi"("error in (no error)"=w782, "Verify GPIB address"=w720, "Instrument type"=enum16{"Supply", "LCR", "Multimeter"}."Multimeter", "Instrument name IN"="Ris Voltmeter") -> ("Instrument name OUT"=w775:string, "Multimeter"=w778:refnum<class "MultimeterControl.lvclass">)  [unwired: 2 in, 4 out]
            n500 = Increment(x=w763) -> (x+1=w762:dbl)
            n501 = local read "X Mapping CB Standard"() -> (w730:string[])
            n502 = Bundle By Name(cluster=w789, "Bias Supply"=w780, "SMU"=w779, "Multimeter"=w778, "Initial Voltage [V]"="Ris Initial Voltage [V]", "Final Voltage [V]"="Ris Final Voltage [V]", "Step Size [V]"="Ris Step Size [V]", "Step Interval [s]"="Ris Step Interval [s]", "Number Of Steps"=w762, "Ramp down steps [V]"="Ris Ramp down steps [V]", "Ramp down Interval [s]"="Ris Ramp down Interval [s]", "Temperature Readout"="Ris Temperature Readout", "Supply Name"=w777, "SMU Name"=w776, "Voltmeter Name"=w775, "R_is Limit [MOhm]"="R_is Limit [MOhm]") -> (w788:T5)
            n503 = Decrement(x=w741) -> (x-1=w743:i32)
            n504 = Decrement(x=w742) -> (x-1=w744:i32)
            n505 = Decrement(x=w725) -> (x-1=w740:i32)
            n506 = Decrement(x=w726) -> (x-1=w721:i32)
            n507 = Decrement(x=w727) -> (x-1=w722:i32)
            n508 = Decrement(x=w724) -> (x-1=w723:i32)
            n509 = Decrement(x=w733) -> (x-1=w735:i32)
            n510 = Decrement(x=w734) -> (x-1=w736:i32)
            n511 = Decrement(x=w731) -> (x-1=w737:i32)
            n512 = Decrement(x=w732) -> (x-1=w738:i32)
            n513 = global write "QC_MeasurementSetup.vi" "Ris Measurement Parameters"(w788) -> ()
            n514 = Replace Array Subset(array=w730, new element #1="SMU LO (GND)" ("Input Element"), index #1=w743, new element #2="SMU HI" ("Input Element"), index #2=w744, new element #3=w739, index #3=w740, new element #4=w739, index #4=w721, new element #5=w739, index #5=w722, new element #6=w739, index #6=w723, new element #7=w739, index #7=w735, new element #8=w739, index #8=w736, new element #9=w739, index #9=w737, new element #10=w739, index #10=w738) -> (w728:string[])
            n515 = local write "X Mapping"(w728) -> ()
          }
          frame "PTP" {
            w799 = ""
            n516 = local read "Y Mapping"() -> (w797:string[])
            n517 = local read "X Mapping CB Standard"() -> (w791:string[])
            n518 = Replace Array Subset(array=w797, new element #1="MUX" ("String"), index #1=0, new element #2="Common GND" ("String"), index #2=1, new element #3=w799, index #3=2, new element #4=w799, index #4=3) -> (w794:string[])
            n519 = local write "X Mapping"(w791) -> ()
            n520 = local write "Y Mapping"(w794) -> ()
          }
        }
        n521 = global write "InstrumentSetup.vi" "Instrument GPIB addresses"(w129) -> ()
        n522 = global write "InstrumentSetup.vi" "Instrument GPIB addresses"(w130) -> ()
        n523 = global write "InstrumentSetup.vi" "Instrument GPIB addresses"(w131) -> ()
      }
      n524 = local write "configured?"(w125) -> ()
    }
  }
